vi "NIMS_NS_fir_halfband.vi"(5 "Function name":string, 6 "Line number":i32, 7 "Number of outputs requested":i32, 8 "error in (no error)":errorcluster, 11 "[A]":variant[](array[variant])) -> (0 "error out":errorcluster, 3 "[funct(A)]":variant[](array[variant]))   [LabVIEW 2017]
uses:
  <vilib>/imath/engines/lvmath/Functions/Error Handling/error.ctl
  <instcachedir>/0/NIMS_RunTimeType_From StrictType (excl LVString)_1019F277F0A747EDBCA0F6C52CA54500.lvgen/NIMS_RunTimeType_From StrictType (excl LVString)_1019F277F0A747EDBCA0F6C52CA54500_000.vi
  <instcachedir>/0/NIMS_Get Row Vector_w Error - Matrix_7ECCFA0649AF47C08F6F0C496599EB01.lvgen/NIMS_Get Row Vector_w Error - Matrix_7ECCFA0649AF47C08F6F0C496599EB01_000.vi
  <instcachedir>/0/NIMS_Get Scalar_w Error_1987D997E87247DDAC16EA23A5E9E4FC.lvgen/NIMS_Get Scalar_w Error_1987D997E87247DDAC16EA23A5E9E4FC_003.vi
  <instcachedir>/0/NIMS_Complex To Real_BE01396FDE034E8E94CEBBA1E368668D.lvgen/NIMS_Complex To Real_BE01396FDE034E8E94CEBBA1E368668D_000.vi
  <instcachedir>/0/NIMS_Get Row Vector_w Error - Matrix_7ECCFA0649AF47C08F6F0C496599EB01.lvgen/NIMS_Get Row Vector_w Error - Matrix_7ECCFA0649AF47C08F6F0C496599EB01_001.vi
  <instcachedir>/0/NIMS_RunTimeType_To Numeric_1CBDAFC4EFAD4045A1DE52278D16738D.lvgen/NIMS_RunTimeType_To Numeric_1CBDAFC4EFAD4045A1DE52278D16738D_000.vi
  <instcachedir>/0/NIMS_Get Scalar_w Error_1987D997E87247DDAC16EA23A5E9E4FC.lvgen/NIMS_Get Scalar_w Error_1987D997E87247DDAC16EA23A5E9E4FC_000.vi
  <vilib>/addons/Digital Filter Design/NI_DigFilter_MathScript.lvlib
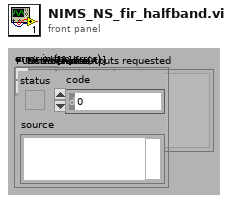
[diagram p1: front panel]
types:
  T1 = typedef "error.ctl" = enum16{"No Error", "Problem", "Input type must not be void", "Incorrect number of parameters", "Function not defined for non-numeric types", "An output variable of the user-defined function is undefined", "Function only defined for character arrays", "Function not defined for boolean, character, or single precision", "Function not defined for complex types", "Not a valid operation", "Inputs must be scalar", "Input matrices are not the same size", "Function only available on RT", "Input matrices must be nonnegative integers of the same type", "Arguments must be non-negative integers less than bitmax", "Number to complement must be less than 2^N", "Bit to get is outside range", "Bit to set is outside range", "Input must be real type ", "At least one parameter must be scalar", "Unable to display plug-in data on RT", "Function not defined for higher dimensional matrices", "Invalid attributes", "Wrong Type of Input Arguments", "Wrong Argument Option", "Invalid file identifier", "Indices must be real positive integers", "The variable is not a matrix data type.", "Number of elements must be the same for indices and values", "You cannot replace elements of a matrix with non-matrix data types.", "Cannot resize a 2D matrix with a linear index", "Unknown variable or symbol", "Indices out of range", "Empty matrix deletion can not be used with two indices", "Number of rows and columns must be the same for indices and values.", "Complex cannot be converted to Boolean", "Char cannot be converted to Boolean", "int64 cannot be converted to Boolean", "uint64 cannot be converted to Boolean", "You cannot convert a Boolean to a character.", "Incompatible input size in 3D surface function", "All rows must have the same number of columns", "Incompatible types", "Invalid matrix dimensions", "Dimension must be 1 or 2", "Base must be an integer between 2 and 36", "Invalid input", "Square matrix required", "Function 'timerstart' must be called before 'timerstop'", "Arguments must be positive real", "Step must not be zero", "Wrong number of input arguments", "Wrong number of output arguments", "Too many index arguments", "Input scalar must be >= 0", "Input scalar must be positive", "Input scalar must not be 0", "Input scalar must be in range [0,1]", "Can't use conditionally defined variable that's undefined", "Input must be a vector", "RT Exec Trace Toolkit not licensed", "Empty vector error", "All elements must be in domain [-1,1]", "All real elements of input vector must be >= 0", "All elements of input vector must be positive", "Values of input vectors are not compatible", "DAQmx not installed", "Input vector must be an increasing vector", "Dereferenced field does not exist within the struct", "A vector or matrix of structures must be indexed before it can be dereferenced", "Lenths of two input vectors are not compatible", "Invalid fieldname", "Empty matrix error", "Cannot use '.' on a type other than Struct", "Unused074", "Data type of the struct's field name is invalid", "Using . to dereference data that is not a struct", "Input struct contains invalid type ", "Size of input matrix is incompatible with input size", "Invalid format specifier", "Could not find field within struct", "Bad permutation array", "Mismatched fieldnames", "ode: User Function could not be opened", "ode: User Function signature does not meet ode requirements", "Unused085", "RunTime: MathScript could not be compiled", "Unknown function", "Only scalars and strings supported", "ode: User Function signature has incorrect number of inputs", "ode:User Function signature has incorrect number of outputs", "Range is too large", "End used without variable", "Function not available (RTE)", "Custom user error", "Arguments must be integers less than bitmax", "Shared library not found", "Header file not found", "Shared library already loaded", "Shared library not loaded", "Shared library function not found", "Shared library string return problem", "Problem calling shared library function", "Problem loading shared library from OS", "Problem parsing shared library header file", "Shared library incompatible types", "Shared library unsupported return type", "Shared library function not exported", "Shared library unsupported input type", "Problem unloading shared library from OS", "Function only available from UI", "Function specified in argument is missing", "An internal error has occurred", "Invalid object", "Invalid property", "Read-only property", "A break command has occurred", "A continue command has occurred", "A return command has occurred", "ode: times parameter invalid", "Function specified in argument has incorrect signature", "Function not found in file", "Reserved keyword cannot be defined as variable", "Reserved keyword cannot be defined as a function or script", "Arguments must be string literals", "Function not supported on this platform", "All columns must have the same number of rows", "Function ignored in RTE warning", "Cannot use : as a parameter that is not a variable", "Output can't be coerced to requested type", "Function not supported on current target", "Variable dependent on an unwired function input", "Unused132", "Unused133", "Unused134", "Unused135", "Unused136", "Unused137", "Unused138", "Unused139", "Global/Persistent must only take constants as arguments.", "Varargin must be last input in the function definition.", "Varargout must be last output in the function definition.", "Invalid output type. Cannot output a cell array of any type other than string.", "Invalid output type. Type is a dynamic struct.", "Invalid output type. Type is a struct that has a field whose type is not known until run-time", "Invalid output type. Type is a struct that has a field which is a plot object.", "MathScript parser DLL missing", "MathScript requires LabVIEW Full", "MathScript license is invalid or missing", "Varargout not supported except in assignments."}
  T2 = typedef "NIMS_CH_character datatype.ctl" = cluster{"Numeric":u8}
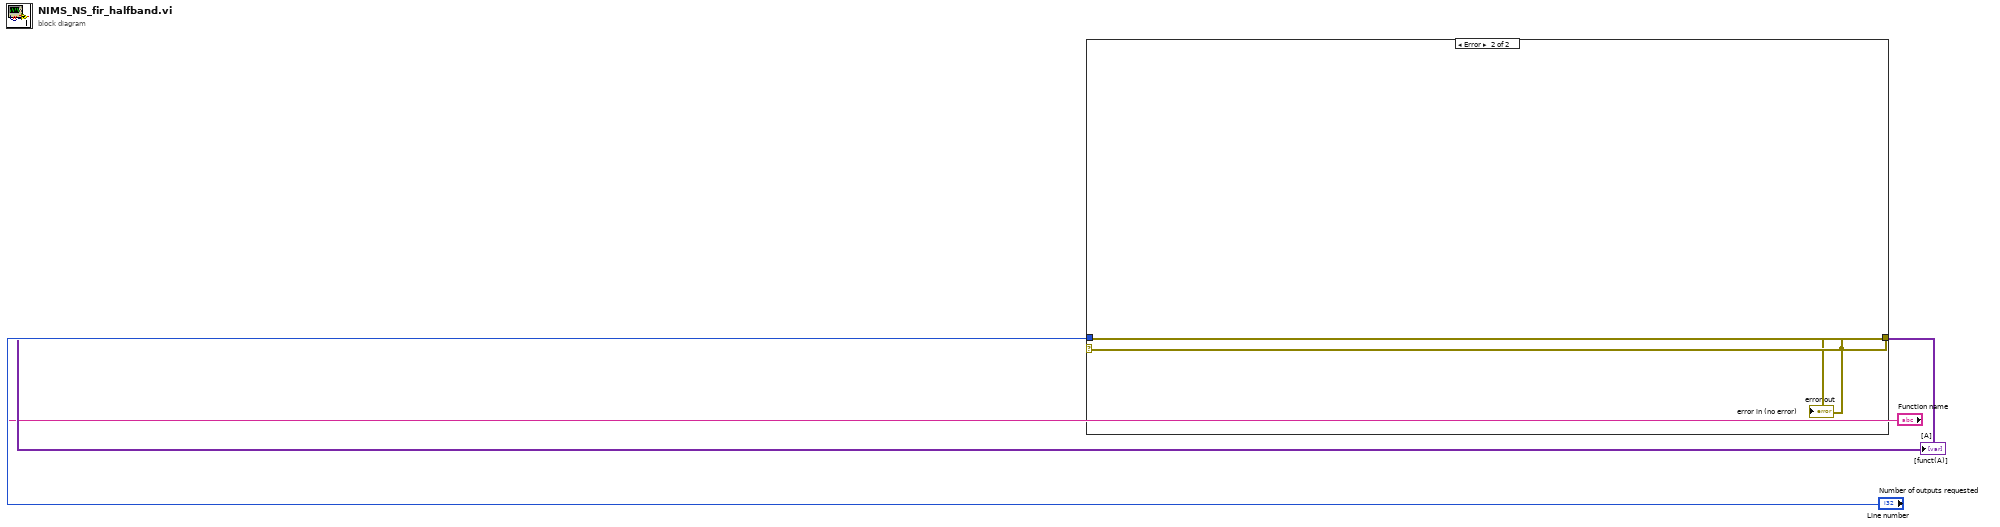
[diagram p0: block diagram]
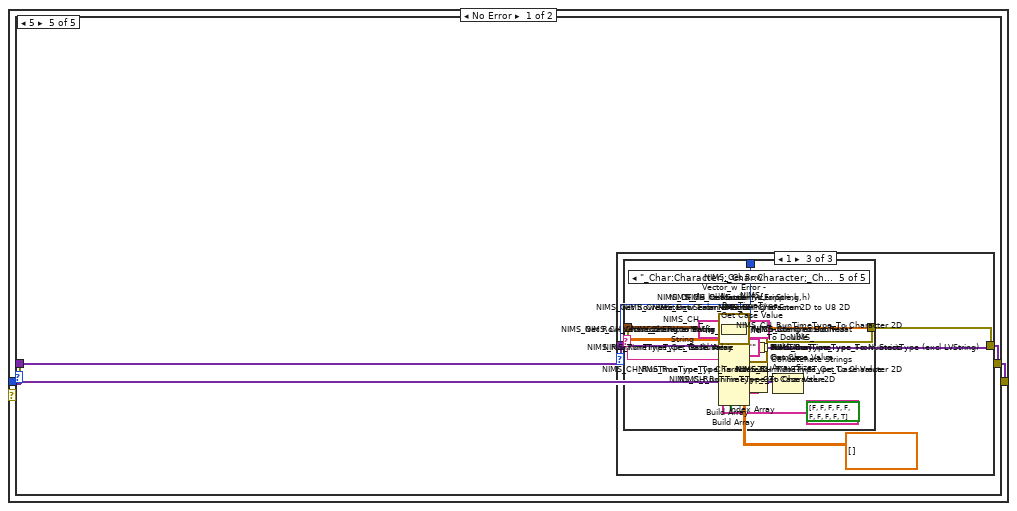
[diagram p2: hidden frame]
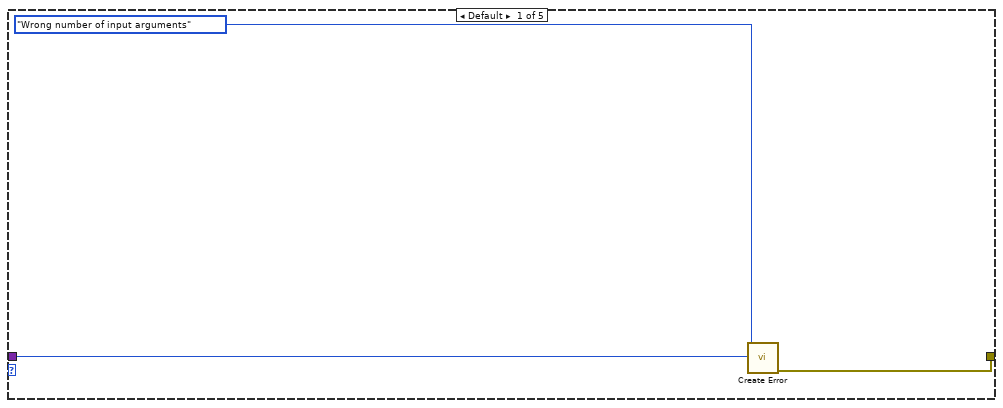
[diagram p3: hidden frame]
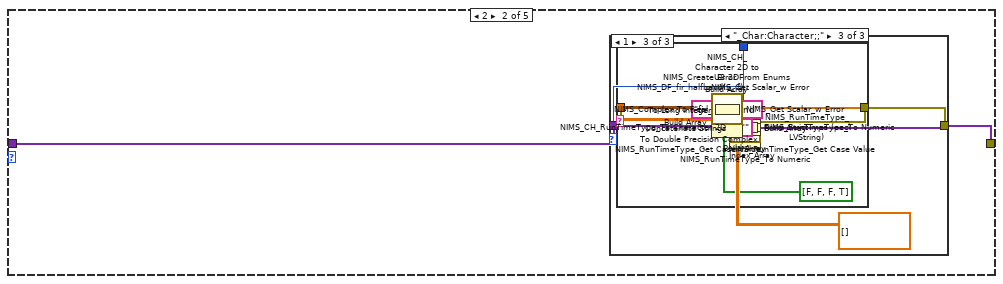
[diagram p4: hidden frame]
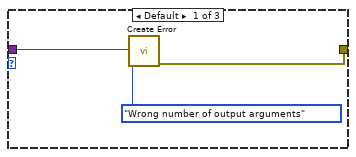
[diagram p5: hidden frame]
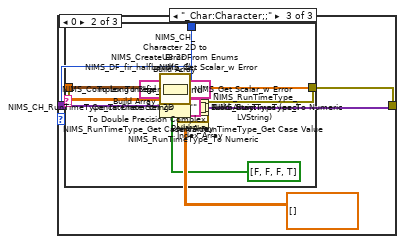
[diagram p6: hidden frame]
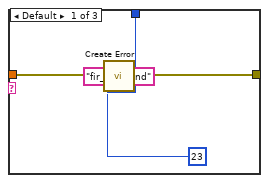
[diagram p7: hidden frame]
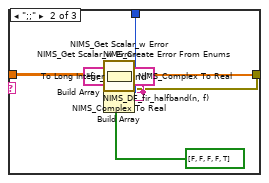
[diagram p8: hidden frame]
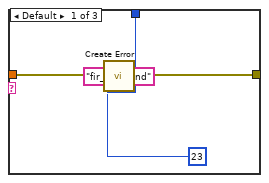
[diagram p9: hidden frame]
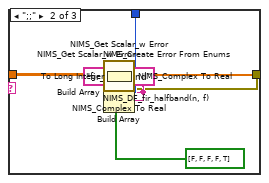
[diagram p10: hidden frame]
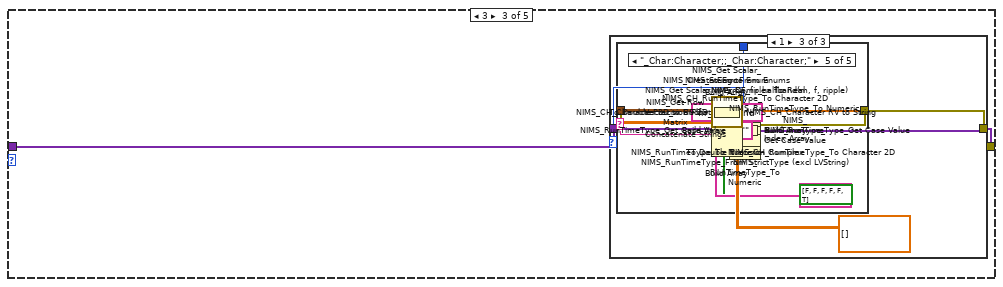
[diagram p11: hidden frame]
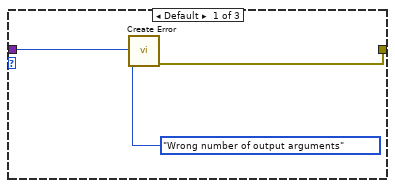
[diagram p12: hidden frame]
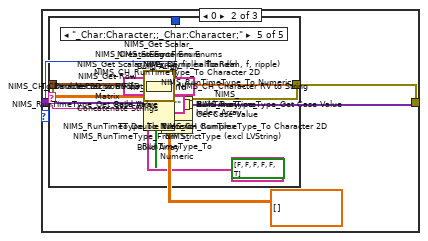
[diagram p13: hidden frame]
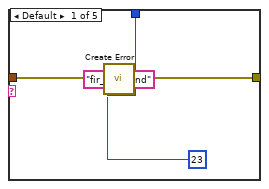
[diagram p14: hidden frame]
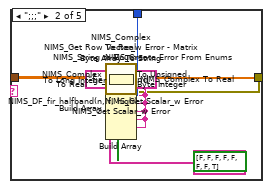
[diagram p15: hidden frame]
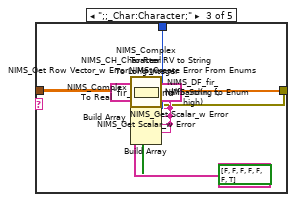
[diagram p16: hidden frame]
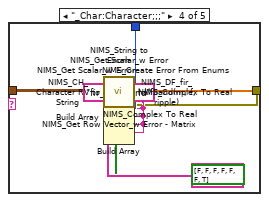
[diagram p17: hidden frame]
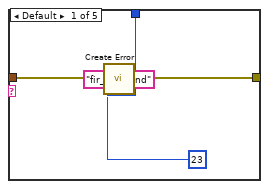
[diagram p18: hidden frame]
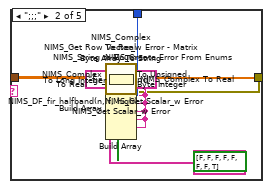
[diagram p19: hidden frame]
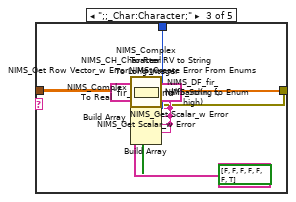
[diagram p20: hidden frame]
diagram:
  n1 = case shown="Error" "error in (no error)" {
    selector: "error in (no error)" -> [_ w1249]
    tunnel: [w15 _] -> w4
    tunnel: [w14 w1249] -> w3
    tunnel: "error in (no error)" -> [w13 _]
    tunnel: "Number of outputs requested" -> [w12 _]
    tunnel: "[A]" -> [w11 _]
    tunnel: "Function name" -> [w10 _]
    tunnel: "Line number" -> [w9 _]
    frame No Error {
      n2 = Array Size(array=w11) -> (size(s)=w8:i32)
      n3 = case shown="5" w8 {
        tunnel: [_ w27 w171 w469 w831] -> w15
        tunnel: w10 -> [w19 w24 w168 w466 w828]
        tunnel: w9 -> [w20 w25 w169 w467 w829]
        tunnel: w13 -> [w17 w23 w167 w465 w827]
        tunnel: [w16 w22 w166 w464 w826] -> w14
        tunnel: w12 -> [_ w21 w165 w463 w825]
        tunnel: w11 -> [_ w26 w170 w468 w830]
        frame Default {
          n4 = call <vilib>:"Create Error.vi"("Function name"=w19, "error in (no error)"=w17, "Error Enum"=error."Wrong number of input arguments", "Line number"=w20) -> ("error out"=w16:errorcluster)  [unwired: 6 in, 1 out]
        }
        frame 2 {
          n5 = case shown="1" w21 {
            tunnel: [_ w33 w99] -> w27
            tunnel: w24 -> [w31 _ _]
            tunnel: w25 -> [w32 w51 w117]
            tunnel: w23 -> [w29 w49 w115]
            tunnel: [w28 w39 w105] -> w22
            tunnel: w26 -> [_ w52 w118]
            frame Default {
              n6 = call <vilib>:"Create Error.vi"("Function name"=w31, "error in (no error)"=w29, "Error Enum"=error."Wrong number of output arguments", "Line number"=w32) -> ("error out"=w28:errorcluster)  [unwired: 6 in, 1 out]
            }
            frame 0 {
              n7 = Index Array(array=w52) -> (element #1=w48:variant, element #2=w43:variant)  [unwired: 2 in]
              n8 = call <vilib>:"NIMS_RunTimeType_Get Case Value.vi"("Data In"=w43) -> ("Case Value"=w40:string)  [unwired: 9 in, 1 out]
              n9 = call-generic <vilib>:"NIMS_RunTimeType_To Numeric.vi"("DataType"=cdb[][] [], "Variant"=w43) -> ("data"=w41:cdb[][])  [unwired: 1 in]
              n10 = call <vilib>:"NIMS_RunTimeType_Get Case Value.vi"("Data In"=w48) -> ("Case Value"=w44:string)  [unwired: 9 in, 1 out]
              n11 = call <vilib>:"NIMS_CH_RunTimeType_To Character 2D.vi"("Variant"=w48) -> ("data"=w45:T2[][])  [unwired: 1 in]
              n12 = call-generic <vilib>:"NIMS_RunTimeType_To Numeric.vi"("DataType"=cdb[][] [], "Variant"=w48) -> ("data"=w46:cdb[][])  [unwired: 1 in]
              n13 = Concatenate Strings(w44, w40) -> (w50:string)
              n14 = case shown="\"_Char:Character;;\"" w50 {
                tunnel: w49 -> [w54 w63 w84]
                tunnel: [_ w58 w79] -> w38
                tunnel: [w53 w59 w80] -> w39
                tunnel: w46 -> [_ w77 _]
                tunnel: w45 -> [_ _ w97]
                tunnel: w41 -> [_ w73 w93]
                tunnel: w51 -> [w57 w66 w87]
                frame Default {
                  n15 = call <vilib>:"Create Error.vi"("Function name"="fir_halfband", "error in (no error)"=w54, "Error Enum"=23, "Line number"=w57) -> ("error out"=w53:errorcluster)  [unwired: 6 in, 1 out]
                }
                frame ";;" {
                  w61 = "fir_halfband"
                  n16 = call-generic <vilib>:"NIMS_Complex To Real.vi"("A"=w73) -> ("Error Enum"=w69:T1, "Real(A)"=w72:dbl[][])  [unwired: 8 in, 1 out]
                  n17 = call-generic <vilib>:"NIMS_Get Scalar_w Error.vi"("A"=w72) -> ("Error Enum"=w68:T1, "Scalar"=w74:dbl)  [unwired: 8 in, 1 out]
                  n18 = call-generic <vilib>:"NIMS_Complex To Real.vi"("A"=w77) -> ("Error Enum"=w71:T1, "Real(A)"=w76:dbl[][])  [unwired: 8 in, 1 out]
                  n19 = To Long Integer(number=w76) -> (32bit integer=w75:i32[][])
                  n20 = call-generic <vilib>:"NIMS_Get Scalar_w Error.vi"("A"=w75) -> ("Error Enum"=w70:T1, "Scalar"=w78:i32)  [unwired: 8 in, 1 out]
                  n21 = call <vilib>:"NIMS_DF_fir_halfband(n, f).vi"("f"=w74, "n"=w78) -> ("error"=w67:i32, "b"=w58:dbl[])  [unwired: 8 in]
                  n22 = Build Array(w61, w61, w61, w61, "fir_halfband") -> (w64:string[])
                  n23 = Build Array(w71, w70, w69, w68, w67) -> (w65:i32[])
                  n24 = call <vilib>:"NIMS_Create Error From Enums.vi"("Error Code"=bool[] [FALSE, FALSE, FALSE, FALSE, TRUE], "error in (no error)"=w63, "Line no"=w66, "Error Enums"=w65, "Function names"=w64) -> ("error out"=w59:errorcluster)  [unwired: 6 in]
                }
                frame "_Char:Character;;" {
                  w82 = "fir_halfband"
                  n25 = call-generic <vilib>:"NIMS_Complex To Real.vi"("A"=w93) -> ("Error Enum"=w90:T1, "Real(A)"=w92:dbl[][])  [unwired: 8 in, 1 out]
                  n26 = call-generic <vilib>:"NIMS_Get Scalar_w Error.vi"("A"=w92) -> ("Error Enum"=w89:T1, "Scalar"=w94:dbl)  [unwired: 8 in, 1 out]
                  n27 = call <vilib>:"NIMS_CH_Character 2D to U8 2D.vi"("Character 2D array"=w97) -> ("U8 2D array"=w96:u8[][])  [unwired: 10 in]
                  n28 = To Long Integer(number=w96) -> (32bit integer=w95:i32[][])
                  n29 = call-generic <vilib>:"NIMS_Get Scalar_w Error.vi"("A"=w95) -> ("Error Enum"=w91:T1, "Scalar"=w98:i32)  [unwired: 8 in, 1 out]
                  n30 = call <vilib>:"NIMS_DF_fir_halfband(n, f).vi"("f"=w94, "n"=w98) -> ("error"=w88:i32, "b"=w79:dbl[])  [unwired: 8 in]
                  n31 = Build Array(w82, w82, w82, "fir_halfband") -> (w85:string[])
                  n32 = Build Array(w91, w90, w89, w88) -> (w86:i32[])
                  n33 = call <vilib>:"NIMS_Create Error From Enums.vi"("Error Code"=bool[] [FALSE, FALSE, FALSE, TRUE], "error in (no error)"=w84, "Line no"=w87, "Error Enums"=w86, "Function names"=w85) -> ("error out"=w80:errorcluster)  [unwired: 6 in]
                }
              }
              n34 = Build Array(w38) -> (w37:dbl[][])
              n35 = To Double Precision Complex(1:w37) -> (0:w36:cdb[][])
              n36 = call-generic <vilib>:"NIMS_RunTimeType_From StrictType (excl LVString).vi"("Plug-In Name"="", "Data In"=w36) -> ("Data Out"=w34:variant)  [unwired: 2 in]
              n37 = Build Array(w34) -> (w33:variant[])
            }
            frame 1 {
              n38 = Index Array(array=w118) -> (element #1=w114:variant, element #2=w109:variant)  [unwired: 2 in]
              n39 = call <vilib>:"NIMS_RunTimeType_Get Case Value.vi"("Data In"=w109) -> ("Case Value"=w106:string)  [unwired: 9 in, 1 out]
              n40 = call-generic <vilib>:"NIMS_RunTimeType_To Numeric.vi"("DataType"=cdb[][] [], "Variant"=w109) -> ("data"=w107:cdb[][])  [unwired: 1 in]
              n41 = call <vilib>:"NIMS_RunTimeType_Get Case Value.vi"("Data In"=w114) -> ("Case Value"=w110:string)  [unwired: 9 in, 1 out]
              n42 = call <vilib>:"NIMS_CH_RunTimeType_To Character 2D.vi"("Variant"=w114) -> ("data"=w111:T2[][])  [unwired: 1 in]
              n43 = call-generic <vilib>:"NIMS_RunTimeType_To Numeric.vi"("DataType"=cdb[][] [], "Variant"=w114) -> ("data"=w112:cdb[][])  [unwired: 1 in]
              n44 = Concatenate Strings(w110, w106) -> (w116:string)
              n45 = case shown="\"_Char:Character;;\"" w116 {
                tunnel: w115 -> [w120 w129 w150]
                tunnel: [_ w124 w145] -> w104
                tunnel: [w119 w125 w146] -> w105
                tunnel: w112 -> [_ w143 _]
                tunnel: w111 -> [_ _ w163]
                tunnel: w107 -> [_ w139 w159]
                tunnel: w117 -> [w123 w132 w153]
                frame Default {
                  n46 = call <vilib>:"Create Error.vi"("Function name"="fir_halfband", "error in (no error)"=w120, "Error Enum"=23, "Line number"=w123) -> ("error out"=w119:errorcluster)  [unwired: 6 in, 1 out]
                }
                frame ";;" {
                  w127 = "fir_halfband"
                  n47 = call-generic <vilib>:"NIMS_Complex To Real.vi"("A"=w139) -> ("Error Enum"=w135:T1, "Real(A)"=w138:dbl[][])  [unwired: 8 in, 1 out]
                  n48 = call-generic <vilib>:"NIMS_Get Scalar_w Error.vi"("A"=w138) -> ("Error Enum"=w134:T1, "Scalar"=w140:dbl)  [unwired: 8 in, 1 out]
                  n49 = call-generic <vilib>:"NIMS_Complex To Real.vi"("A"=w143) -> ("Error Enum"=w137:T1, "Real(A)"=w142:dbl[][])  [unwired: 8 in, 1 out]
                  n50 = To Long Integer(number=w142) -> (32bit integer=w141:i32[][])
                  n51 = call-generic <vilib>:"NIMS_Get Scalar_w Error.vi"("A"=w141) -> ("Error Enum"=w136:T1, "Scalar"=w144:i32)  [unwired: 8 in, 1 out]
                  n52 = call <vilib>:"NIMS_DF_fir_halfband(n, f).vi"("f"=w140, "n"=w144) -> ("error"=w133:i32, "b"=w124:dbl[])  [unwired: 8 in]
                  n53 = Build Array(w127, w127, w127, w127, "fir_halfband") -> (w130:string[])
                  n54 = Build Array(w137, w136, w135, w134, w133) -> (w131:i32[])
                  n55 = call <vilib>:"NIMS_Create Error From Enums.vi"("Error Code"=bool[] [FALSE, FALSE, FALSE, FALSE, TRUE], "error in (no error)"=w129, "Line no"=w132, "Error Enums"=w131, "Function names"=w130) -> ("error out"=w125:errorcluster)  [unwired: 6 in]
                }
                frame "_Char:Character;;" {
                  w148 = "fir_halfband"
                  n56 = call-generic <vilib>:"NIMS_Complex To Real.vi"("A"=w159) -> ("Error Enum"=w156:T1, "Real(A)"=w158:dbl[][])  [unwired: 8 in, 1 out]
                  n57 = call-generic <vilib>:"NIMS_Get Scalar_w Error.vi"("A"=w158) -> ("Error Enum"=w155:T1, "Scalar"=w160:dbl)  [unwired: 8 in, 1 out]
                  n58 = call <vilib>:"NIMS_CH_Character 2D to U8 2D.vi"("Character 2D array"=w163) -> ("U8 2D array"=w162:u8[][])  [unwired: 10 in]
                  n59 = To Long Integer(number=w162) -> (32bit integer=w161:i32[][])
                  n60 = call-generic <vilib>:"NIMS_Get Scalar_w Error.vi"("A"=w161) -> ("Error Enum"=w157:T1, "Scalar"=w164:i32)  [unwired: 8 in, 1 out]
                  n61 = call <vilib>:"NIMS_DF_fir_halfband(n, f).vi"("f"=w160, "n"=w164) -> ("error"=w154:i32, "b"=w145:dbl[])  [unwired: 8 in]
                  n62 = Build Array(w148, w148, w148, "fir_halfband") -> (w151:string[])
                  n63 = Build Array(w157, w156, w155, w154) -> (w152:i32[])
                  n64 = call <vilib>:"NIMS_Create Error From Enums.vi"("Error Code"=bool[] [FALSE, FALSE, FALSE, TRUE], "error in (no error)"=w150, "Line no"=w153, "Error Enums"=w152, "Function names"=w151) -> ("error out"=w146:errorcluster)  [unwired: 6 in]
                }
              }
              n65 = Build Array(w104) -> (w103:dbl[][])
              n66 = To Double Precision Complex(1:w103) -> (0:w102:cdb[][])
              n67 = call-generic <vilib>:"NIMS_RunTimeType_From StrictType (excl LVString).vi"("Plug-In Name"="", "Data In"=w102) -> ("Data Out"=w100:variant)  [unwired: 2 in]
              n68 = Build Array(w100) -> (w99:variant[])
            }
          }
        }
        frame 3 {
          n69 = case shown="1" w165 {
            tunnel: [_ w177 w320] -> w171
            tunnel: w168 -> [w175 _ _]
            tunnel: w169 -> [w176 w200 w343]
            tunnel: w167 -> [w173 w198 w341]
            tunnel: [w172 w183 w326] -> w166
            tunnel: w170 -> [_ w201 w344]
            frame Default {
              n70 = call <vilib>:"Create Error.vi"("Function name"=w175, "error in (no error)"=w173, "Error Enum"=error."Wrong number of output arguments", "Line number"=w176) -> ("error out"=w172:errorcluster)  [unwired: 6 in, 1 out]
            }
            frame 0 {
              n71 = Index Array(array=w201) -> (element #1=w197:variant, element #2=w192:variant, element #3=w188:variant)  [unwired: 3 in]
              n72 = call <vilib>:"NIMS_RunTimeType_Get Case Value.vi"("Data In"=w188) -> ("Case Value"=w184:string)  [unwired: 9 in, 1 out]
              n73 = call <vilib>:"NIMS_CH_RunTimeType_To Character 2D.vi"("Variant"=w188) -> ("data"=w185:T2[][])  [unwired: 1 in]
              n74 = call-generic <vilib>:"NIMS_RunTimeType_To Numeric.vi"("DataType"=cdb[][] [], "Variant"=w188) -> ("data"=w186:cdb[][])  [unwired: 1 in]
              n75 = call <vilib>:"NIMS_RunTimeType_Get Case Value.vi"("Data In"=w192) -> ("Case Value"=w189:string)  [unwired: 9 in, 1 out]
              n76 = call-generic <vilib>:"NIMS_RunTimeType_To Numeric.vi"("DataType"=cdb[][] [], "Variant"=w192) -> ("data"=w190:cdb[][])  [unwired: 1 in]
              n77 = call <vilib>:"NIMS_RunTimeType_Get Case Value.vi"("Data In"=w197) -> ("Case Value"=w193:string)  [unwired: 9 in, 1 out]
              n78 = call <vilib>:"NIMS_CH_RunTimeType_To Character 2D.vi"("Variant"=w197) -> ("data"=w194:T2[][])  [unwired: 1 in]
              n79 = call-generic <vilib>:"NIMS_RunTimeType_To Numeric.vi"("DataType"=cdb[][] [], "Variant"=w197) -> ("data"=w195:cdb[][])  [unwired: 1 in]
              n80 = Concatenate Strings(w193, w189, w184) -> (w199:string)
              n81 = case shown="\"_Char:Character;;_Char:Character;\"" w199 {
                tunnel: w198 -> [w203 w212 w243 w271 w298]
                tunnel: [_ w207 w238 w266 w293] -> w182
                tunnel: [w202 w208 w239 w267 w294] -> w183
                tunnel: w195 -> [_ w236 w264 _ _]
                tunnel: w194 -> [_ _ _ w290 w317]
                tunnel: w190 -> [_ w232 w260 w286 w313]
                tunnel: w186 -> [_ w228 _ w283 _]
                tunnel: w185 -> [_ _ w256 _ w310]
                tunnel: w200 -> [w206 w215 w246 w274 w301]
                frame Default {
                  n82 = call <vilib>:"Create Error.vi"("Function name"="fir_halfband", "error in (no error)"=w203, "Error Enum"=23, "Line number"=w206) -> ("error out"=w202:errorcluster)  [unwired: 6 in, 1 out]
                }
                frame ";;;" {
                  w210 = "fir_halfband"
                  n83 = call-generic <vilib>:"NIMS_Complex To Real.vi"("A"=w228) -> ("Error Enum"=w219:T1, "Real(A)"=w227:dbl[][])  [unwired: 8 in, 1 out]
                  n84 = To Unsigned Byte Integer(number=w227) -> (unsigned 8bit integer=w226:u8[][])
                  n85 = call-generic <vilib>:"NIMS_Get Row Vector_w Error - Matrix.vi"("A"=w226) -> ("Error Enum"=w218:T1, "Row Vector"=w225:u8[])  [unwired: 8 in, 1 out]
                  n86 = Byte Array To String(unsigned byte array=w225) -> (string=w229:string)
                  n87 = call <vilib>:"NIMS_String to Enum.vi"("Input String"=w229, "Enum choices"=string[] ["high"] ("Enum Options")) -> ("Error Enum"=w217:T1, "Enum Index"=w230:i32)  [unwired: 8 in]
                  n88 = call-generic <vilib>:"NIMS_Complex To Real.vi"("A"=w232) -> ("Error Enum"=w221:T1, "Real(A)"=w231:dbl[][])  [unwired: 8 in, 1 out]
                  n89 = call-generic <vilib>:"NIMS_Get Scalar_w Error.vi"("A"=w231) -> ("Error Enum"=w220:T1, "Scalar"=w233:dbl)  [unwired: 8 in, 1 out]
                  n90 = call-generic <vilib>:"NIMS_Complex To Real.vi"("A"=w236) -> ("Error Enum"=w223:T1, "Real(A)"=w235:dbl[][])  [unwired: 8 in, 1 out]
                  n91 = To Long Integer(number=w235) -> (32bit integer=w234:i32[][])
                  n92 = call-generic <vilib>:"NIMS_Get Scalar_w Error.vi"("A"=w234) -> ("Error Enum"=w222:T1, "Scalar"=w237:i32)  [unwired: 8 in, 1 out]
                  n93 = call <vilib>:"NIMS_DF_fir_halfband(n, f, high).vi"("type"=w230, "f"=w233, "n"=w237) -> ("error"=w216:i32, "b"=w207:dbl[])  [unwired: 7 in]
                  n94 = Build Array(w210, w210, w210, w210, w210, w210, w210, "fir_halfband") -> (w213:string[])
                  n95 = Build Array(w223, w222, w221, w220, w219, w218, w217, w216) -> (w214:i32[])
                  n96 = call <vilib>:"NIMS_Create Error From Enums.vi"("Error Code"=bool[] [FALSE, FALSE, FALSE, FALSE, FALSE, FALSE, FALSE, TRUE], "error in (no error)"=w212, "Line no"=w215, "Error Enums"=w214, "Function names"=w213) -> ("error out"=w208:errorcluster)  [unwired: 6 in]
                }
                frame ";;_Char:Character;" {
                  w241 = "fir_halfband"
                  n97 = call-generic <vilib>:"NIMS_Get Row Vector_w Error - Matrix.vi"("A"=w256) -> ("Error Enum"=w249:T1, "Row Vector"=w255:T2[])  [unwired: 8 in, 1 out]
                  n98 = call <vilib>:"NIMS_CH_Character RV to String.vi"("Character array"=w255) -> ("String"=w257:string)  [unwired: 10 in]
                  n99 = call <vilib>:"NIMS_String to Enum.vi"("Input String"=w257, "Enum choices"=string[] ["high"] ("Enum Options")) -> ("Error Enum"=w248:T1, "Enum Index"=w258:i32)  [unwired: 8 in]
                  n100 = call-generic <vilib>:"NIMS_Complex To Real.vi"("A"=w260) -> ("Error Enum"=w251:T1, "Real(A)"=w259:dbl[][])  [unwired: 8 in, 1 out]
                  n101 = call-generic <vilib>:"NIMS_Get Scalar_w Error.vi"("A"=w259) -> ("Error Enum"=w250:T1, "Scalar"=w261:dbl)  [unwired: 8 in, 1 out]
                  n102 = call-generic <vilib>:"NIMS_Complex To Real.vi"("A"=w264) -> ("Error Enum"=w253:T1, "Real(A)"=w263:dbl[][])  [unwired: 8 in, 1 out]
                  n103 = To Long Integer(number=w263) -> (32bit integer=w262:i32[][])
                  n104 = call-generic <vilib>:"NIMS_Get Scalar_w Error.vi"("A"=w262) -> ("Error Enum"=w252:T1, "Scalar"=w265:i32)  [unwired: 8 in, 1 out]
                  n105 = call <vilib>:"NIMS_DF_fir_halfband(n, f, high).vi"("type"=w258, "f"=w261, "n"=w265) -> ("error"=w247:i32, "b"=w238:dbl[])  [unwired: 7 in]
                  n106 = Build Array(w241, w241, w241, w241, w241, w241, "fir_halfband") -> (w244:string[])
                  n107 = Build Array(w253, w252, w251, w250, w249, w248, w247) -> (w245:i32[])
                  n108 = call <vilib>:"NIMS_Create Error From Enums.vi"("Error Code"=bool[] [FALSE, FALSE, FALSE, FALSE, FALSE, FALSE, TRUE], "error in (no error)"=w243, "Line no"=w246, "Error Enums"=w245, "Function names"=w244) -> ("error out"=w239:errorcluster)  [unwired: 6 in]
                }
                frame "_Char:Character;;;" {
                  w269 = "fir_halfband"
                  n109 = call-generic <vilib>:"NIMS_Complex To Real.vi"("A"=w283) -> ("Error Enum"=w277:T1, "Real(A)"=w282:dbl[][])  [unwired: 8 in, 1 out]
                  n110 = call-generic <vilib>:"NIMS_Get Scalar_w Error.vi"("A"=w282) -> ("Error Enum"=w276:T1, "Scalar"=w284:dbl)  [unwired: 8 in, 1 out]
                  n111 = call-generic <vilib>:"NIMS_Complex To Real.vi"("A"=w286) -> ("Error Enum"=w279:T1, "Real(A)"=w285:dbl[][])  [unwired: 8 in, 1 out]
                  n112 = call-generic <vilib>:"NIMS_Get Scalar_w Error.vi"("A"=w285) -> ("Error Enum"=w278:T1, "Scalar"=w287:dbl)  [unwired: 8 in, 1 out]
                  n113 = call-generic <vilib>:"NIMS_Get Row Vector_w Error - Matrix.vi"("A"=w290) -> ("Error Enum"=w281:T1, "Row Vector"=w289:T2[])  [unwired: 8 in, 1 out]
                  n114 = call <vilib>:"NIMS_CH_Character RV to String.vi"("Character array"=w289) -> ("String"=w291:string)  [unwired: 10 in]
                  n115 = call <vilib>:"NIMS_String to Enum.vi"("Input String"=w291, "Enum choices"=string[] ["minorder"] ("Enum Options")) -> ("Error Enum"=w280:T1, "Enum Index"=w292:i32)  [unwired: 8 in]
                  n116 = call <vilib>:"NIMS_DF_fir_halfband(m, f, ripple).vi"("ripple"=w284, "f"=w287, "flag"=w292) -> ("error"=w275:i32, "b"=w266:dbl[])  [unwired: 7 in]
                  n117 = Build Array(w269, w269, w269, w269, w269, w269, "fir_halfband") -> (w272:string[])
                  n118 = Build Array(w281, w280, w279, w278, w277, w276, w275) -> (w273:i32[])
                  n119 = call <vilib>:"NIMS_Create Error From Enums.vi"("Error Code"=bool[] [FALSE, FALSE, FALSE, FALSE, FALSE, FALSE, TRUE], "error in (no error)"=w271, "Line no"=w274, "Error Enums"=w273, "Function names"=w272) -> ("error out"=w267:errorcluster)  [unwired: 6 in]
                }
                frame "_Char:Character;;_Char:Character;" {
                  w296 = "fir_halfband"
                  n120 = call <vilib>:"NIMS_CH_Character 2D to U8 2D.vi"("Character 2D array"=w310) -> ("U8 2D array"=w309:u8[][])  [unwired: 10 in]
                  n121 = To Double Precision Float(number=w309) -> (double precision float=w308:dbl[][])
                  n122 = call-generic <vilib>:"NIMS_Get Scalar_w Error.vi"("A"=w308) -> ("Error Enum"=w303:T1, "Scalar"=w311:dbl)  [unwired: 8 in, 1 out]
                  n123 = call-generic <vilib>:"NIMS_Complex To Real.vi"("A"=w313) -> ("Error Enum"=w305:T1, "Real(A)"=w312:dbl[][])  [unwired: 8 in, 1 out]
                  n124 = call-generic <vilib>:"NIMS_Get Scalar_w Error.vi"("A"=w312) -> ("Error Enum"=w304:T1, "Scalar"=w314:dbl)  [unwired: 8 in, 1 out]
                  n125 = call-generic <vilib>:"NIMS_Get Row Vector_w Error - Matrix.vi"("A"=w317) -> ("Error Enum"=w307:T1, "Row Vector"=w316:T2[])  [unwired: 8 in, 1 out]
                  n126 = call <vilib>:"NIMS_CH_Character RV to String.vi"("Character array"=w316) -> ("String"=w318:string)  [unwired: 10 in]
                  n127 = call <vilib>:"NIMS_String to Enum.vi"("Input String"=w318, "Enum choices"=string[] ["minorder"] ("Enum Options")) -> ("Error Enum"=w306:T1, "Enum Index"=w319:i32)  [unwired: 8 in]
                  n128 = call <vilib>:"NIMS_DF_fir_halfband(m, f, ripple).vi"("ripple"=w311, "f"=w314, "flag"=w319) -> ("error"=w302:i32, "b"=w293:dbl[])  [unwired: 7 in]
                  n129 = Build Array(w296, w296, w296, w296, w296, "fir_halfband") -> (w299:string[])
                  n130 = Build Array(w307, w306, w305, w304, w303, w302) -> (w300:i32[])
                  n131 = call <vilib>:"NIMS_Create Error From Enums.vi"("Error Code"=bool[] [FALSE, FALSE, FALSE, FALSE, FALSE, TRUE], "error in (no error)"=w298, "Line no"=w301, "Error Enums"=w300, "Function names"=w299) -> ("error out"=w294:errorcluster)  [unwired: 6 in]
                }
              }
              n132 = Build Array(w182) -> (w181:dbl[][])
              n133 = To Double Precision Complex(1:w181) -> (0:w180:cdb[][])
              n134 = call-generic <vilib>:"NIMS_RunTimeType_From StrictType (excl LVString).vi"("Plug-In Name"="", "Data In"=w180) -> ("Data Out"=w178:variant)  [unwired: 2 in]
              n135 = Build Array(w178) -> (w177:variant[])
            }
            frame 1 {
              n136 = Index Array(array=w344) -> (element #1=w340:variant, element #2=w335:variant, element #3=w331:variant)  [unwired: 3 in]
              n137 = call <vilib>:"NIMS_RunTimeType_Get Case Value.vi"("Data In"=w331) -> ("Case Value"=w327:string)  [unwired: 9 in, 1 out]
              n138 = call <vilib>:"NIMS_CH_RunTimeType_To Character 2D.vi"("Variant"=w331) -> ("data"=w328:T2[][])  [unwired: 1 in]
              n139 = call-generic <vilib>:"NIMS_RunTimeType_To Numeric.vi"("DataType"=cdb[][] [], "Variant"=w331) -> ("data"=w329:cdb[][])  [unwired: 1 in]
              n140 = call <vilib>:"NIMS_RunTimeType_Get Case Value.vi"("Data In"=w335) -> ("Case Value"=w332:string)  [unwired: 9 in, 1 out]
              n141 = call-generic <vilib>:"NIMS_RunTimeType_To Numeric.vi"("DataType"=cdb[][] [], "Variant"=w335) -> ("data"=w333:cdb[][])  [unwired: 1 in]
              n142 = call <vilib>:"NIMS_RunTimeType_Get Case Value.vi"("Data In"=w340) -> ("Case Value"=w336:string)  [unwired: 9 in, 1 out]
              n143 = call <vilib>:"NIMS_CH_RunTimeType_To Character 2D.vi"("Variant"=w340) -> ("data"=w337:T2[][])  [unwired: 1 in]
              n144 = call-generic <vilib>:"NIMS_RunTimeType_To Numeric.vi"("DataType"=cdb[][] [], "Variant"=w340) -> ("data"=w338:cdb[][])  [unwired: 1 in]
              n145 = Concatenate Strings(w336, w332, w327) -> (w342:string)
              n146 = case shown="\"_Char:Character;;_Char:Character;\"" w342 {
                tunnel: w341 -> [w346 w355 w386 w414 w441]
                tunnel: [_ w350 w381 w409 w436] -> w325
                tunnel: [w345 w351 w382 w410 w437] -> w326
                tunnel: w338 -> [_ w379 w407 _ _]
                tunnel: w337 -> [_ _ _ w433 w460]
                tunnel: w333 -> [_ w375 w403 w429 w456]
                tunnel: w329 -> [_ w371 _ w426 _]
                tunnel: w328 -> [_ _ w399 _ w453]
                tunnel: w343 -> [w349 w358 w389 w417 w444]
                frame Default {
                  n147 = call <vilib>:"Create Error.vi"("Function name"="fir_halfband", "error in (no error)"=w346, "Error Enum"=23, "Line number"=w349) -> ("error out"=w345:errorcluster)  [unwired: 6 in, 1 out]
                }
                frame ";;;" {
                  w353 = "fir_halfband"
                  n148 = call-generic <vilib>:"NIMS_Complex To Real.vi"("A"=w371) -> ("Error Enum"=w362:T1, "Real(A)"=w370:dbl[][])  [unwired: 8 in, 1 out]
                  n149 = To Unsigned Byte Integer(number=w370) -> (unsigned 8bit integer=w369:u8[][])
                  n150 = call-generic <vilib>:"NIMS_Get Row Vector_w Error - Matrix.vi"("A"=w369) -> ("Error Enum"=w361:T1, "Row Vector"=w368:u8[])  [unwired: 8 in, 1 out]
                  n151 = Byte Array To String(unsigned byte array=w368) -> (string=w372:string)
                  n152 = call <vilib>:"NIMS_String to Enum.vi"("Input String"=w372, "Enum choices"=string[] ["high"] ("Enum Options")) -> ("Error Enum"=w360:T1, "Enum Index"=w373:i32)  [unwired: 8 in]
                  n153 = call-generic <vilib>:"NIMS_Complex To Real.vi"("A"=w375) -> ("Error Enum"=w364:T1, "Real(A)"=w374:dbl[][])  [unwired: 8 in, 1 out]
                  n154 = call-generic <vilib>:"NIMS_Get Scalar_w Error.vi"("A"=w374) -> ("Error Enum"=w363:T1, "Scalar"=w376:dbl)  [unwired: 8 in, 1 out]
                  n155 = call-generic <vilib>:"NIMS_Complex To Real.vi"("A"=w379) -> ("Error Enum"=w366:T1, "Real(A)"=w378:dbl[][])  [unwired: 8 in, 1 out]
                  n156 = To Long Integer(number=w378) -> (32bit integer=w377:i32[][])
                  n157 = call-generic <vilib>:"NIMS_Get Scalar_w Error.vi"("A"=w377) -> ("Error Enum"=w365:T1, "Scalar"=w380:i32)  [unwired: 8 in, 1 out]
                  n158 = call <vilib>:"NIMS_DF_fir_halfband(n, f, high).vi"("type"=w373, "f"=w376, "n"=w380) -> ("error"=w359:i32, "b"=w350:dbl[])  [unwired: 7 in]
                  n159 = Build Array(w353, w353, w353, w353, w353, w353, w353, "fir_halfband") -> (w356:string[])
                  n160 = Build Array(w366, w365, w364, w363, w362, w361, w360, w359) -> (w357:i32[])
                  n161 = call <vilib>:"NIMS_Create Error From Enums.vi"("Error Code"=bool[] [FALSE, FALSE, FALSE, FALSE, FALSE, FALSE, FALSE, TRUE], "error in (no error)"=w355, "Line no"=w358, "Error Enums"=w357, "Function names"=w356) -> ("error out"=w351:errorcluster)  [unwired: 6 in]
                }
                frame ";;_Char:Character;" {
                  w384 = "fir_halfband"
                  n162 = call-generic <vilib>:"NIMS_Get Row Vector_w Error - Matrix.vi"("A"=w399) -> ("Error Enum"=w392:T1, "Row Vector"=w398:T2[])  [unwired: 8 in, 1 out]
                  n163 = call <vilib>:"NIMS_CH_Character RV to String.vi"("Character array"=w398) -> ("String"=w400:string)  [unwired: 10 in]
                  n164 = call <vilib>:"NIMS_String to Enum.vi"("Input String"=w400, "Enum choices"=string[] ["high"] ("Enum Options")) -> ("Error Enum"=w391:T1, "Enum Index"=w401:i32)  [unwired: 8 in]
                  n165 = call-generic <vilib>:"NIMS_Complex To Real.vi"("A"=w403) -> ("Error Enum"=w394:T1, "Real(A)"=w402:dbl[][])  [unwired: 8 in, 1 out]
                  n166 = call-generic <vilib>:"NIMS_Get Scalar_w Error.vi"("A"=w402) -> ("Error Enum"=w393:T1, "Scalar"=w404:dbl)  [unwired: 8 in, 1 out]
                  n167 = call-generic <vilib>:"NIMS_Complex To Real.vi"("A"=w407) -> ("Error Enum"=w396:T1, "Real(A)"=w406:dbl[][])  [unwired: 8 in, 1 out]
                  n168 = To Long Integer(number=w406) -> (32bit integer=w405:i32[][])
                  n169 = call-generic <vilib>:"NIMS_Get Scalar_w Error.vi"("A"=w405) -> ("Error Enum"=w395:T1, "Scalar"=w408:i32)  [unwired: 8 in, 1 out]
                  n170 = call <vilib>:"NIMS_DF_fir_halfband(n, f, high).vi"("type"=w401, "f"=w404, "n"=w408) -> ("error"=w390:i32, "b"=w381:dbl[])  [unwired: 7 in]
                  n171 = Build Array(w384, w384, w384, w384, w384, w384, "fir_halfband") -> (w387:string[])
                  n172 = Build Array(w396, w395, w394, w393, w392, w391, w390) -> (w388:i32[])
                  n173 = call <vilib>:"NIMS_Create Error From Enums.vi"("Error Code"=bool[] [FALSE, FALSE, FALSE, FALSE, FALSE, FALSE, TRUE], "error in (no error)"=w386, "Line no"=w389, "Error Enums"=w388, "Function names"=w387) -> ("error out"=w382:errorcluster)  [unwired: 6 in]
                }
                frame "_Char:Character;;;" {
                  w412 = "fir_halfband"
                  n174 = call-generic <vilib>:"NIMS_Complex To Real.vi"("A"=w426) -> ("Error Enum"=w420:T1, "Real(A)"=w425:dbl[][])  [unwired: 8 in, 1 out]
                  n175 = call-generic <vilib>:"NIMS_Get Scalar_w Error.vi"("A"=w425) -> ("Error Enum"=w419:T1, "Scalar"=w427:dbl)  [unwired: 8 in, 1 out]
                  n176 = call-generic <vilib>:"NIMS_Complex To Real.vi"("A"=w429) -> ("Error Enum"=w422:T1, "Real(A)"=w428:dbl[][])  [unwired: 8 in, 1 out]
                  n177 = call-generic <vilib>:"NIMS_Get Scalar_w Error.vi"("A"=w428) -> ("Error Enum"=w421:T1, "Scalar"=w430:dbl)  [unwired: 8 in, 1 out]
                  n178 = call-generic <vilib>:"NIMS_Get Row Vector_w Error - Matrix.vi"("A"=w433) -> ("Error Enum"=w424:T1, "Row Vector"=w432:T2[])  [unwired: 8 in, 1 out]
                  n179 = call <vilib>:"NIMS_CH_Character RV to String.vi"("Character array"=w432) -> ("String"=w434:string)  [unwired: 10 in]
                  n180 = call <vilib>:"NIMS_String to Enum.vi"("Input String"=w434, "Enum choices"=string[] ["minorder"] ("Enum Options")) -> ("Error Enum"=w423:T1, "Enum Index"=w435:i32)  [unwired: 8 in]
                  n181 = call <vilib>:"NIMS_DF_fir_halfband(m, f, ripple).vi"("ripple"=w427, "f"=w430, "flag"=w435) -> ("error"=w418:i32, "b"=w409:dbl[])  [unwired: 7 in]
                  n182 = Build Array(w412, w412, w412, w412, w412, w412, "fir_halfband") -> (w415:string[])
                  n183 = Build Array(w424, w423, w422, w421, w420, w419, w418) -> (w416:i32[])
                  n184 = call <vilib>:"NIMS_Create Error From Enums.vi"("Error Code"=bool[] [FALSE, FALSE, FALSE, FALSE, FALSE, FALSE, TRUE], "error in (no error)"=w414, "Line no"=w417, "Error Enums"=w416, "Function names"=w415) -> ("error out"=w410:errorcluster)  [unwired: 6 in]
                }
                frame "_Char:Character;;_Char:Character;" {
                  w439 = "fir_halfband"
                  n185 = call <vilib>:"NIMS_CH_Character 2D to U8 2D.vi"("Character 2D array"=w453) -> ("U8 2D array"=w452:u8[][])  [unwired: 10 in]
                  n186 = To Double Precision Float(number=w452) -> (double precision float=w451:dbl[][])
                  n187 = call-generic <vilib>:"NIMS_Get Scalar_w Error.vi"("A"=w451) -> ("Error Enum"=w446:T1, "Scalar"=w454:dbl)  [unwired: 8 in, 1 out]
                  n188 = call-generic <vilib>:"NIMS_Complex To Real.vi"("A"=w456) -> ("Error Enum"=w448:T1, "Real(A)"=w455:dbl[][])  [unwired: 8 in, 1 out]
                  n189 = call-generic <vilib>:"NIMS_Get Scalar_w Error.vi"("A"=w455) -> ("Error Enum"=w447:T1, "Scalar"=w457:dbl)  [unwired: 8 in, 1 out]
                  n190 = call-generic <vilib>:"NIMS_Get Row Vector_w Error - Matrix.vi"("A"=w460) -> ("Error Enum"=w450:T1, "Row Vector"=w459:T2[])  [unwired: 8 in, 1 out]
                  n191 = call <vilib>:"NIMS_CH_Character RV to String.vi"("Character array"=w459) -> ("String"=w461:string)  [unwired: 10 in]
                  n192 = call <vilib>:"NIMS_String to Enum.vi"("Input String"=w461, "Enum choices"=string[] ["minorder"] ("Enum Options")) -> ("Error Enum"=w449:T1, "Enum Index"=w462:i32)  [unwired: 8 in]
                  n193 = call <vilib>:"NIMS_DF_fir_halfband(m, f, ripple).vi"("ripple"=w454, "f"=w457, "flag"=w462) -> ("error"=w445:i32, "b"=w436:dbl[])  [unwired: 7 in]
                  n194 = Build Array(w439, w439, w439, w439, w439, "fir_halfband") -> (w442:string[])
                  n195 = Build Array(w450, w449, w448, w447, w446, w445) -> (w443:i32[])
                  n196 = call <vilib>:"NIMS_Create Error From Enums.vi"("Error Code"=bool[] [FALSE, FALSE, FALSE, FALSE, FALSE, TRUE], "error in (no error)"=w441, "Line no"=w444, "Error Enums"=w443, "Function names"=w442) -> ("error out"=w437:errorcluster)  [unwired: 6 in]
                }
              }
              n197 = Build Array(w325) -> (w324:dbl[][])
              n198 = To Double Precision Complex(1:w324) -> (0:w323:cdb[][])
              n199 = call-generic <vilib>:"NIMS_RunTimeType_From StrictType (excl LVString).vi"("Plug-In Name"="", "Data In"=w323) -> ("Data Out"=w321:variant)  [unwired: 2 in]
              n200 = Build Array(w321) -> (w320:variant[])
            }
          }
        }
        frame 4 {
          n201 = case shown="1" w463 {
            tunnel: [_ w475 w650] -> w469
            tunnel: w466 -> [w473 _ _]
            tunnel: w467 -> [w474 w501 w676]
            tunnel: w465 -> [w471 w499 w674]
            tunnel: [w470 w481 w656] -> w464
            tunnel: w468 -> [_ w502 w677]
            frame Default {
              n202 = call <vilib>:"Create Error.vi"("Function name"=w473, "error in (no error)"=w471, "Error Enum"=error."Wrong number of output arguments", "Line number"=w474) -> ("error out"=w470:errorcluster)  [unwired: 6 in, 1 out]
            }
            frame 0 {
              n203 = Index Array(array=w502) -> (element #1=w498:variant, element #2=w493:variant, element #3=w489:variant, element #4=w484:variant)  [unwired: 4 in]
              n204 = call <vilib>:"NIMS_RunTimeType_Get Case Value.vi"("Data In"=w484) -> ("Case Value"=w482:string)  [unwired: 9 in, 1 out]
              n205 = call <vilib>:"NIMS_CH_RunTimeType_To Character 2D.vi"("Variant"=w484) -> ("data"=w483:T2[][])  [unwired: 1 in]
              n206 = call <vilib>:"NIMS_RunTimeType_Get Case Value.vi"("Data In"=w489) -> ("Case Value"=w485:string)  [unwired: 9 in, 1 out]
              n207 = call <vilib>:"NIMS_CH_RunTimeType_To Character 2D.vi"("Variant"=w489) -> ("data"=w486:T2[][])  [unwired: 1 in]
              n208 = call-generic <vilib>:"NIMS_RunTimeType_To Numeric.vi"("DataType"=cdb[][] [], "Variant"=w489) -> ("data"=w487:cdb[][])  [unwired: 1 in]
              n209 = call <vilib>:"NIMS_RunTimeType_Get Case Value.vi"("Data In"=w493) -> ("Case Value"=w490:string)  [unwired: 9 in, 1 out]
              n210 = call-generic <vilib>:"NIMS_RunTimeType_To Numeric.vi"("DataType"=cdb[][] [], "Variant"=w493) -> ("data"=w491:cdb[][])  [unwired: 1 in]
              n211 = call <vilib>:"NIMS_RunTimeType_Get Case Value.vi"("Data In"=w498) -> ("Case Value"=w494:string)  [unwired: 9 in, 1 out]
              n212 = call <vilib>:"NIMS_CH_RunTimeType_To Character 2D.vi"("Variant"=w498) -> ("data"=w495:T2[][])  [unwired: 1 in]
              n213 = call-generic <vilib>:"NIMS_RunTimeType_To Numeric.vi"("DataType"=cdb[][] [], "Variant"=w498) -> ("data"=w496:cdb[][])  [unwired: 1 in]
              n214 = Concatenate Strings(w494, w490, w485, w482) -> (w500:string)
              n215 = case shown="\"_Char:Character;;_Char:Character;_Char:Character;\"" w500 {
                tunnel: w499 -> [w504 w513 w550 w587 w621]
                tunnel: [_ w508 w545 w582 w616] -> w480
                tunnel: [w503 w509 w546 w583 w617] -> w481
                tunnel: w496 -> [_ w542 w579 _ _]
                tunnel: w495 -> [_ _ _ w613 w647]
                tunnel: w491 -> [_ w536 w573 w609 w643]
                tunnel: w487 -> [_ w533 _ w606 _]
                tunnel: w486 -> [_ _ w570 _ w640]
                tunnel: w483 -> [_ w529 w565 w602 w635]
                tunnel: w501 -> [w507 w516 w553 w590 w624]
                frame Default {
                  n216 = call <vilib>:"Create Error.vi"("Function name"="fir_halfband", "error in (no error)"=w504, "Error Enum"=23, "Line number"=w507) -> ("error out"=w503:errorcluster)  [unwired: 6 in, 1 out]
                }
                frame ";;;_Char:Character;" {
                  w511 = "fir_halfband"
                  n217 = call-generic <vilib>:"NIMS_Get Row Vector_w Error - Matrix.vi"("A"=w529) -> ("Error Enum"=w519:T1, "Row Vector"=w528:T2[])  [unwired: 8 in, 1 out]
                  n218 = call <vilib>:"NIMS_CH_Character RV to String.vi"("Character array"=w528) -> ("String"=w530:string)  [unwired: 10 in]
                  n219 = call <vilib>:"NIMS_String to Enum.vi"("Input String"=w530, "Enum choices"=string[] ["high", "kaiser"] ("Enum Options")) -> ("Error Enum"=w518:T1, "Enum Index"=w531:i32)  [unwired: 8 in]
                  n220 = call-generic <vilib>:"NIMS_Complex To Real.vi"("A"=w533) -> ("Error Enum"=w521:T1, "Real(A)"=w532:dbl[][])  [unwired: 8 in, 1 out]
                  n221 = call-generic <vilib>:"NIMS_Get Scalar_w Error.vi"("A"=w532) -> ("Error Enum"=w520:T1, "Scalar"=w534:dbl)  [unwired: 8 in, 1 out]
                  n222 = call-generic <vilib>:"NIMS_Complex To Real.vi"("A"=w536) -> ("Error Enum"=w523:T1, "Real(A)"=w535:dbl[][])  [unwired: 8 in, 1 out]
                  n223 = call-generic <vilib>:"NIMS_Get Scalar_w Error.vi"("A"=w535) -> ("Error Enum"=w522:T1, "Scalar"=w537:dbl)  [unwired: 8 in, 1 out]
                  n224 = call-generic <vilib>:"NIMS_Complex To Real.vi"("A"=w542) -> ("Error Enum"=w526:T1, "Real(A)"=w541:dbl[][])  [unwired: 8 in, 1 out]
                  n225 = To Unsigned Byte Integer(number=w541) -> (unsigned 8bit integer=w540:u8[][])
                  n226 = call-generic <vilib>:"NIMS_Get Row Vector_w Error - Matrix.vi"("A"=w540) -> ("Error Enum"=w525:T1, "Row Vector"=w539:u8[])  [unwired: 8 in, 1 out]
                  n227 = Byte Array To String(unsigned byte array=w539) -> (string=w543:string)
                  n228 = call <vilib>:"NIMS_String to Enum.vi"("Input String"=w543, "Enum choices"=string[] ["minorder"] ("Enum Options")) -> ("Error Enum"=w524:T1, "Enum Index"=w544:i32)  [unwired: 8 in]
                  n229 = call <vilib>:"NIMS_DF_fir_halfband(m, f, ripple,kh).vi"("type"=w531, "ripple"=w534, "f"=w537, "flag"=w544) -> ("error"=w517:i32, "b"=w508:dbl[])  [unwired: 6 in]
                  n230 = Build Array(w511, w511, w511, w511, w511, w511, w511, w511, w511, "fir_halfband") -> (w514:string[])
                  n231 = Build Array(w526, w525, w524, w523, w522, w521, w520, w519, w518, w517) -> (w515:i32[])
                  n232 = call <vilib>:"NIMS_Create Error From Enums.vi"("Error Code"=bool[] [FALSE, FALSE, FALSE, FALSE, FALSE, FALSE, FALSE, FALSE, FALSE, TRUE], "error in (no error)"=w513, "Line no"=w516, "Error Enums"=w515, "Function names"=w514) -> ("error out"=w509:errorcluster)  [unwired: 6 in]
                }
                frame ";;_Char:Character;_Char:Character;" {
                  w548 = "fir_halfband"
                  n233 = call-generic <vilib>:"NIMS_Get Row Vector_w Error - Matrix.vi"("A"=w565) -> ("Error Enum"=w556:T1, "Row Vector"=w564:T2[])  [unwired: 8 in, 1 out]
                  n234 = call <vilib>:"NIMS_CH_Character RV to String.vi"("Character array"=w564) -> ("String"=w566:string)  [unwired: 10 in]
                  n235 = call <vilib>:"NIMS_String to Enum.vi"("Input String"=w566, "Enum choices"=string[] ["high", "kaiser"] ("Enum Options")) -> ("Error Enum"=w555:T1, "Enum Index"=w567:i32)  [unwired: 8 in]
                  n236 = call <vilib>:"NIMS_CH_Character 2D to U8 2D.vi"("Character 2D array"=w570) -> ("U8 2D array"=w569:u8[][])  [unwired: 10 in]
                  n237 = To Double Precision Float(number=w569) -> (double precision float=w568:dbl[][])
                  n238 = call-generic <vilib>:"NIMS_Get Scalar_w Error.vi"("A"=w568) -> ("Error Enum"=w557:T1, "Scalar"=w571:dbl)  [unwired: 8 in, 1 out]
                  n239 = call-generic <vilib>:"NIMS_Complex To Real.vi"("A"=w573) -> ("Error Enum"=w559:T1, "Real(A)"=w572:dbl[][])  [unwired: 8 in, 1 out]
                  n240 = call-generic <vilib>:"NIMS_Get Scalar_w Error.vi"("A"=w572) -> ("Error Enum"=w558:T1, "Scalar"=w574:dbl)  [unwired: 8 in, 1 out]
                  n241 = call-generic <vilib>:"NIMS_Complex To Real.vi"("A"=w579) -> ("Error Enum"=w562:T1, "Real(A)"=w578:dbl[][])  [unwired: 8 in, 1 out]
                  n242 = To Unsigned Byte Integer(number=w578) -> (unsigned 8bit integer=w577:u8[][])
                  n243 = call-generic <vilib>:"NIMS_Get Row Vector_w Error - Matrix.vi"("A"=w577) -> ("Error Enum"=w561:T1, "Row Vector"=w576:u8[])  [unwired: 8 in, 1 out]
                  n244 = Byte Array To String(unsigned byte array=w576) -> (string=w580:string)
                  n245 = call <vilib>:"NIMS_String to Enum.vi"("Input String"=w580, "Enum choices"=string[] ["minorder"] ("Enum Options")) -> ("Error Enum"=w560:T1, "Enum Index"=w581:i32)  [unwired: 8 in]
                  n246 = call <vilib>:"NIMS_DF_fir_halfband(m, f, ripple,kh).vi"("type"=w567, "ripple"=w571, "f"=w574, "flag"=w581) -> ("error"=w554:i32, "b"=w545:dbl[])  [unwired: 6 in]
                  n247 = Build Array(w548, w548, w548, w548, w548, w548, w548, w548, "fir_halfband") -> (w551:string[])
                  n248 = Build Array(w562, w561, w560, w559, w558, w557, w556, w555, w554) -> (w552:i32[])
                  n249 = call <vilib>:"NIMS_Create Error From Enums.vi"("Error Code"=bool[] [FALSE, FALSE, FALSE, FALSE, FALSE, FALSE, FALSE, FALSE, TRUE], "error in (no error)"=w550, "Line no"=w553, "Error Enums"=w552, "Function names"=w551) -> ("error out"=w546:errorcluster)  [unwired: 6 in]
                }
                frame "_Char:Character;;;_Char:Character;" {
                  w585 = "fir_halfband"
                  n250 = call-generic <vilib>:"NIMS_Get Row Vector_w Error - Matrix.vi"("A"=w602) -> ("Error Enum"=w593:T1, "Row Vector"=w601:T2[])  [unwired: 8 in, 1 out]
                  n251 = call <vilib>:"NIMS_CH_Character RV to String.vi"("Character array"=w601) -> ("String"=w603:string)  [unwired: 10 in]
                  n252 = call <vilib>:"NIMS_String to Enum.vi"("Input String"=w603, "Enum choices"=string[] ["high", "kaiser"] ("Enum Options")) -> ("Error Enum"=w592:T1, "Enum Index"=w604:i32)  [unwired: 8 in]
                  n253 = call-generic <vilib>:"NIMS_Complex To Real.vi"("A"=w606) -> ("Error Enum"=w595:T1, "Real(A)"=w605:dbl[][])  [unwired: 8 in, 1 out]
                  n254 = call-generic <vilib>:"NIMS_Get Scalar_w Error.vi"("A"=w605) -> ("Error Enum"=w594:T1, "Scalar"=w607:dbl)  [unwired: 8 in, 1 out]
                  n255 = call-generic <vilib>:"NIMS_Complex To Real.vi"("A"=w609) -> ("Error Enum"=w597:T1, "Real(A)"=w608:dbl[][])  [unwired: 8 in, 1 out]
                  n256 = call-generic <vilib>:"NIMS_Get Scalar_w Error.vi"("A"=w608) -> ("Error Enum"=w596:T1, "Scalar"=w610:dbl)  [unwired: 8 in, 1 out]
                  n257 = call-generic <vilib>:"NIMS_Get Row Vector_w Error - Matrix.vi"("A"=w613) -> ("Error Enum"=w599:T1, "Row Vector"=w612:T2[])  [unwired: 8 in, 1 out]
                  n258 = call <vilib>:"NIMS_CH_Character RV to String.vi"("Character array"=w612) -> ("String"=w614:string)  [unwired: 10 in]
                  n259 = call <vilib>:"NIMS_String to Enum.vi"("Input String"=w614, "Enum choices"=string[] ["minorder"] ("Enum Options")) -> ("Error Enum"=w598:T1, "Enum Index"=w615:i32)  [unwired: 8 in]
                  n260 = call <vilib>:"NIMS_DF_fir_halfband(m, f, ripple,kh).vi"("type"=w604, "ripple"=w607, "f"=w610, "flag"=w615) -> ("error"=w591:i32, "b"=w582:dbl[])  [unwired: 6 in]
                  n261 = Build Array(w585, w585, w585, w585, w585, w585, w585, w585, "fir_halfband") -> (w588:string[])
                  n262 = Build Array(w599, w598, w597, w596, w595, w594, w593, w592, w591) -> (w589:i32[])
                  n263 = call <vilib>:"NIMS_Create Error From Enums.vi"("Error Code"=bool[] [FALSE, FALSE, FALSE, FALSE, FALSE, FALSE, FALSE, FALSE, TRUE], "error in (no error)"=w587, "Line no"=w590, "Error Enums"=w589, "Function names"=w588) -> ("error out"=w583:errorcluster)  [unwired: 6 in]
                }
                frame "_Char:Character;;_Char:Character;_Char:Character;" {
                  w619 = "fir_halfband"
                  n264 = call-generic <vilib>:"NIMS_Get Row Vector_w Error - Matrix.vi"("A"=w635) -> ("Error Enum"=w627:T1, "Row Vector"=w634:T2[])  [unwired: 8 in, 1 out]
                  n265 = call <vilib>:"NIMS_CH_Character RV to String.vi"("Character array"=w634) -> ("String"=w636:string)  [unwired: 10 in]
                  n266 = call <vilib>:"NIMS_String to Enum.vi"("Input String"=w636, "Enum choices"=string[] ["high", "kaiser"] ("Enum Options")) -> ("Error Enum"=w626:T1, "Enum Index"=w637:i32)  [unwired: 8 in]
                  n267 = call <vilib>:"NIMS_CH_Character 2D to U8 2D.vi"("Character 2D array"=w640) -> ("U8 2D array"=w639:u8[][])  [unwired: 10 in]
                  n268 = To Double Precision Float(number=w639) -> (double precision float=w638:dbl[][])
                  n269 = call-generic <vilib>:"NIMS_Get Scalar_w Error.vi"("A"=w638) -> ("Error Enum"=w628:T1, "Scalar"=w641:dbl)  [unwired: 8 in, 1 out]
                  n270 = call-generic <vilib>:"NIMS_Complex To Real.vi"("A"=w643) -> ("Error Enum"=w630:T1, "Real(A)"=w642:dbl[][])  [unwired: 8 in, 1 out]
                  n271 = call-generic <vilib>:"NIMS_Get Scalar_w Error.vi"("A"=w642) -> ("Error Enum"=w629:T1, "Scalar"=w644:dbl)  [unwired: 8 in, 1 out]
                  n272 = call-generic <vilib>:"NIMS_Get Row Vector_w Error - Matrix.vi"("A"=w647) -> ("Error Enum"=w632:T1, "Row Vector"=w646:T2[])  [unwired: 8 in, 1 out]
                  n273 = call <vilib>:"NIMS_CH_Character RV to String.vi"("Character array"=w646) -> ("String"=w648:string)  [unwired: 10 in]
                  n274 = call <vilib>:"NIMS_String to Enum.vi"("Input String"=w648, "Enum choices"=string[] ["minorder"] ("Enum Options")) -> ("Error Enum"=w631:T1, "Enum Index"=w649:i32)  [unwired: 8 in]
                  n275 = call <vilib>:"NIMS_DF_fir_halfband(m, f, ripple,kh).vi"("type"=w637, "ripple"=w641, "f"=w644, "flag"=w649) -> ("error"=w625:i32, "b"=w616:dbl[])  [unwired: 6 in]
                  n276 = Build Array(w619, w619, w619, w619, w619, w619, w619, "fir_halfband") -> (w622:string[])
                  n277 = Build Array(w632, w631, w630, w629, w628, w627, w626, w625) -> (w623:i32[])
                  n278 = call <vilib>:"NIMS_Create Error From Enums.vi"("Error Code"=bool[] [FALSE, FALSE, FALSE, FALSE, FALSE, FALSE, FALSE, TRUE], "error in (no error)"=w621, "Line no"=w624, "Error Enums"=w623, "Function names"=w622) -> ("error out"=w617:errorcluster)  [unwired: 6 in]
                }
              }
              n279 = Build Array(w480) -> (w479:dbl[][])
              n280 = To Double Precision Complex(1:w479) -> (0:w478:cdb[][])
              n281 = call-generic <vilib>:"NIMS_RunTimeType_From StrictType (excl LVString).vi"("Plug-In Name"="", "Data In"=w478) -> ("Data Out"=w476:variant)  [unwired: 2 in]
              n282 = Build Array(w476) -> (w475:variant[])
            }
            frame 1 {
              n283 = Index Array(array=w677) -> (element #1=w673:variant, element #2=w668:variant, element #3=w664:variant, element #4=w659:variant)  [unwired: 4 in]
              n284 = call <vilib>:"NIMS_RunTimeType_Get Case Value.vi"("Data In"=w659) -> ("Case Value"=w657:string)  [unwired: 9 in, 1 out]
              n285 = call <vilib>:"NIMS_CH_RunTimeType_To Character 2D.vi"("Variant"=w659) -> ("data"=w658:T2[][])  [unwired: 1 in]
              n286 = call <vilib>:"NIMS_RunTimeType_Get Case Value.vi"("Data In"=w664) -> ("Case Value"=w660:string)  [unwired: 9 in, 1 out]
              n287 = call <vilib>:"NIMS_CH_RunTimeType_To Character 2D.vi"("Variant"=w664) -> ("data"=w661:T2[][])  [unwired: 1 in]
              n288 = call-generic <vilib>:"NIMS_RunTimeType_To Numeric.vi"("DataType"=cdb[][] [], "Variant"=w664) -> ("data"=w662:cdb[][])  [unwired: 1 in]
              n289 = call <vilib>:"NIMS_RunTimeType_Get Case Value.vi"("Data In"=w668) -> ("Case Value"=w665:string)  [unwired: 9 in, 1 out]
              n290 = call-generic <vilib>:"NIMS_RunTimeType_To Numeric.vi"("DataType"=cdb[][] [], "Variant"=w668) -> ("data"=w666:cdb[][])  [unwired: 1 in]
              n291 = call <vilib>:"NIMS_RunTimeType_Get Case Value.vi"("Data In"=w673) -> ("Case Value"=w669:string)  [unwired: 9 in, 1 out]
              n292 = call <vilib>:"NIMS_CH_RunTimeType_To Character 2D.vi"("Variant"=w673) -> ("data"=w670:T2[][])  [unwired: 1 in]
              n293 = call-generic <vilib>:"NIMS_RunTimeType_To Numeric.vi"("DataType"=cdb[][] [], "Variant"=w673) -> ("data"=w671:cdb[][])  [unwired: 1 in]
              n294 = Concatenate Strings(w669, w665, w660, w657) -> (w675:string)
              n295 = case shown="\"_Char:Character;;_Char:Character;_Char:Character;\"" w675 {
                tunnel: w674 -> [w679 w688 w725 w762 w796]
                tunnel: [_ w683 w720 w757 w791] -> w655
                tunnel: [w678 w684 w721 w758 w792] -> w656
                tunnel: w671 -> [_ w717 w754 _ _]
                tunnel: w670 -> [_ _ _ w788 w822]
                tunnel: w666 -> [_ w711 w748 w784 w818]
                tunnel: w662 -> [_ w708 _ w781 _]
                tunnel: w661 -> [_ _ w745 _ w815]
                tunnel: w658 -> [_ w704 w740 w777 w810]
                tunnel: w676 -> [w682 w691 w728 w765 w799]
                frame Default {
                  n296 = call <vilib>:"Create Error.vi"("Function name"="fir_halfband", "error in (no error)"=w679, "Error Enum"=23, "Line number"=w682) -> ("error out"=w678:errorcluster)  [unwired: 6 in, 1 out]
                }
                frame ";;;_Char:Character;" {
                  w686 = "fir_halfband"
                  n297 = call-generic <vilib>:"NIMS_Get Row Vector_w Error - Matrix.vi"("A"=w704) -> ("Error Enum"=w694:T1, "Row Vector"=w703:T2[])  [unwired: 8 in, 1 out]
                  n298 = call <vilib>:"NIMS_CH_Character RV to String.vi"("Character array"=w703) -> ("String"=w705:string)  [unwired: 10 in]
                  n299 = call <vilib>:"NIMS_String to Enum.vi"("Input String"=w705, "Enum choices"=string[] ["high", "kaiser"] ("Enum Options")) -> ("Error Enum"=w693:T1, "Enum Index"=w706:i32)  [unwired: 8 in]
                  n300 = call-generic <vilib>:"NIMS_Complex To Real.vi"("A"=w708) -> ("Error Enum"=w696:T1, "Real(A)"=w707:dbl[][])  [unwired: 8 in, 1 out]
                  n301 = call-generic <vilib>:"NIMS_Get Scalar_w Error.vi"("A"=w707) -> ("Error Enum"=w695:T1, "Scalar"=w709:dbl)  [unwired: 8 in, 1 out]
                  n302 = call-generic <vilib>:"NIMS_Complex To Real.vi"("A"=w711) -> ("Error Enum"=w698:T1, "Real(A)"=w710:dbl[][])  [unwired: 8 in, 1 out]
                  n303 = call-generic <vilib>:"NIMS_Get Scalar_w Error.vi"("A"=w710) -> ("Error Enum"=w697:T1, "Scalar"=w712:dbl)  [unwired: 8 in, 1 out]
                  n304 = call-generic <vilib>:"NIMS_Complex To Real.vi"("A"=w717) -> ("Error Enum"=w701:T1, "Real(A)"=w716:dbl[][])  [unwired: 8 in, 1 out]
                  n305 = To Unsigned Byte Integer(number=w716) -> (unsigned 8bit integer=w715:u8[][])
                  n306 = call-generic <vilib>:"NIMS_Get Row Vector_w Error - Matrix.vi"("A"=w715) -> ("Error Enum"=w700:T1, "Row Vector"=w714:u8[])  [unwired: 8 in, 1 out]
                  n307 = Byte Array To String(unsigned byte array=w714) -> (string=w718:string)
                  n308 = call <vilib>:"NIMS_String to Enum.vi"("Input String"=w718, "Enum choices"=string[] ["minorder"] ("Enum Options")) -> ("Error Enum"=w699:T1, "Enum Index"=w719:i32)  [unwired: 8 in]
                  n309 = call <vilib>:"NIMS_DF_fir_halfband(m, f, ripple,kh).vi"("type"=w706, "ripple"=w709, "f"=w712, "flag"=w719) -> ("error"=w692:i32, "b"=w683:dbl[])  [unwired: 6 in]
                  n310 = Build Array(w686, w686, w686, w686, w686, w686, w686, w686, w686, "fir_halfband") -> (w689:string[])
                  n311 = Build Array(w701, w700, w699, w698, w697, w696, w695, w694, w693, w692) -> (w690:i32[])
                  n312 = call <vilib>:"NIMS_Create Error From Enums.vi"("Error Code"=bool[] [FALSE, FALSE, FALSE, FALSE, FALSE, FALSE, FALSE, FALSE, FALSE, TRUE], "error in (no error)"=w688, "Line no"=w691, "Error Enums"=w690, "Function names"=w689) -> ("error out"=w684:errorcluster)  [unwired: 6 in]
                }
                frame ";;_Char:Character;_Char:Character;" {
                  w723 = "fir_halfband"
                  n313 = call-generic <vilib>:"NIMS_Get Row Vector_w Error - Matrix.vi"("A"=w740) -> ("Error Enum"=w731:T1, "Row Vector"=w739:T2[])  [unwired: 8 in, 1 out]
                  n314 = call <vilib>:"NIMS_CH_Character RV to String.vi"("Character array"=w739) -> ("String"=w741:string)  [unwired: 10 in]
                  n315 = call <vilib>:"NIMS_String to Enum.vi"("Input String"=w741, "Enum choices"=string[] ["high", "kaiser"] ("Enum Options")) -> ("Error Enum"=w730:T1, "Enum Index"=w742:i32)  [unwired: 8 in]
                  n316 = call <vilib>:"NIMS_CH_Character 2D to U8 2D.vi"("Character 2D array"=w745) -> ("U8 2D array"=w744:u8[][])  [unwired: 10 in]
                  n317 = To Double Precision Float(number=w744) -> (double precision float=w743:dbl[][])
                  n318 = call-generic <vilib>:"NIMS_Get Scalar_w Error.vi"("A"=w743) -> ("Error Enum"=w732:T1, "Scalar"=w746:dbl)  [unwired: 8 in, 1 out]
                  n319 = call-generic <vilib>:"NIMS_Complex To Real.vi"("A"=w748) -> ("Error Enum"=w734:T1, "Real(A)"=w747:dbl[][])  [unwired: 8 in, 1 out]
                  n320 = call-generic <vilib>:"NIMS_Get Scalar_w Error.vi"("A"=w747) -> ("Error Enum"=w733:T1, "Scalar"=w749:dbl)  [unwired: 8 in, 1 out]
                  n321 = call-generic <vilib>:"NIMS_Complex To Real.vi"("A"=w754) -> ("Error Enum"=w737:T1, "Real(A)"=w753:dbl[][])  [unwired: 8 in, 1 out]
                  n322 = To Unsigned Byte Integer(number=w753) -> (unsigned 8bit integer=w752:u8[][])
                  n323 = call-generic <vilib>:"NIMS_Get Row Vector_w Error - Matrix.vi"("A"=w752) -> ("Error Enum"=w736:T1, "Row Vector"=w751:u8[])  [unwired: 8 in, 1 out]
                  n324 = Byte Array To String(unsigned byte array=w751) -> (string=w755:string)
                  n325 = call <vilib>:"NIMS_String to Enum.vi"("Input String"=w755, "Enum choices"=string[] ["minorder"] ("Enum Options")) -> ("Error Enum"=w735:T1, "Enum Index"=w756:i32)  [unwired: 8 in]
                  n326 = call <vilib>:"NIMS_DF_fir_halfband(m, f, ripple,kh).vi"("type"=w742, "ripple"=w746, "f"=w749, "flag"=w756) -> ("error"=w729:i32, "b"=w720:dbl[])  [unwired: 6 in]
                  n327 = Build Array(w723, w723, w723, w723, w723, w723, w723, w723, "fir_halfband") -> (w726:string[])
                  n328 = Build Array(w737, w736, w735, w734, w733, w732, w731, w730, w729) -> (w727:i32[])
                  n329 = call <vilib>:"NIMS_Create Error From Enums.vi"("Error Code"=bool[] [FALSE, FALSE, FALSE, FALSE, FALSE, FALSE, FALSE, FALSE, TRUE], "error in (no error)"=w725, "Line no"=w728, "Error Enums"=w727, "Function names"=w726) -> ("error out"=w721:errorcluster)  [unwired: 6 in]
                }
                frame "_Char:Character;;;_Char:Character;" {
                  w760 = "fir_halfband"
                  n330 = call-generic <vilib>:"NIMS_Get Row Vector_w Error - Matrix.vi"("A"=w777) -> ("Error Enum"=w768:T1, "Row Vector"=w776:T2[])  [unwired: 8 in, 1 out]
                  n331 = call <vilib>:"NIMS_CH_Character RV to String.vi"("Character array"=w776) -> ("String"=w778:string)  [unwired: 10 in]
                  n332 = call <vilib>:"NIMS_String to Enum.vi"("Input String"=w778, "Enum choices"=string[] ["high", "kaiser"] ("Enum Options")) -> ("Error Enum"=w767:T1, "Enum Index"=w779:i32)  [unwired: 8 in]
                  n333 = call-generic <vilib>:"NIMS_Complex To Real.vi"("A"=w781) -> ("Error Enum"=w770:T1, "Real(A)"=w780:dbl[][])  [unwired: 8 in, 1 out]
                  n334 = call-generic <vilib>:"NIMS_Get Scalar_w Error.vi"("A"=w780) -> ("Error Enum"=w769:T1, "Scalar"=w782:dbl)  [unwired: 8 in, 1 out]
                  n335 = call-generic <vilib>:"NIMS_Complex To Real.vi"("A"=w784) -> ("Error Enum"=w772:T1, "Real(A)"=w783:dbl[][])  [unwired: 8 in, 1 out]
                  n336 = call-generic <vilib>:"NIMS_Get Scalar_w Error.vi"("A"=w783) -> ("Error Enum"=w771:T1, "Scalar"=w785:dbl)  [unwired: 8 in, 1 out]
                  n337 = call-generic <vilib>:"NIMS_Get Row Vector_w Error - Matrix.vi"("A"=w788) -> ("Error Enum"=w774:T1, "Row Vector"=w787:T2[])  [unwired: 8 in, 1 out]
                  n338 = call <vilib>:"NIMS_CH_Character RV to String.vi"("Character array"=w787) -> ("String"=w789:string)  [unwired: 10 in]
                  n339 = call <vilib>:"NIMS_String to Enum.vi"("Input String"=w789, "Enum choices"=string[] ["minorder"] ("Enum Options")) -> ("Error Enum"=w773:T1, "Enum Index"=w790:i32)  [unwired: 8 in]
                  n340 = call <vilib>:"NIMS_DF_fir_halfband(m, f, ripple,kh).vi"("type"=w779, "ripple"=w782, "f"=w785, "flag"=w790) -> ("error"=w766:i32, "b"=w757:dbl[])  [unwired: 6 in]
                  n341 = Build Array(w760, w760, w760, w760, w760, w760, w760, w760, "fir_halfband") -> (w763:string[])
                  n342 = Build Array(w774, w773, w772, w771, w770, w769, w768, w767, w766) -> (w764:i32[])
                  n343 = call <vilib>:"NIMS_Create Error From Enums.vi"("Error Code"=bool[] [FALSE, FALSE, FALSE, FALSE, FALSE, FALSE, FALSE, FALSE, TRUE], "error in (no error)"=w762, "Line no"=w765, "Error Enums"=w764, "Function names"=w763) -> ("error out"=w758:errorcluster)  [unwired: 6 in]
                }
                frame "_Char:Character;;_Char:Character;_Char:Character;" {
                  w794 = "fir_halfband"
                  n344 = call-generic <vilib>:"NIMS_Get Row Vector_w Error - Matrix.vi"("A"=w810) -> ("Error Enum"=w802:T1, "Row Vector"=w809:T2[])  [unwired: 8 in, 1 out]
                  n345 = call <vilib>:"NIMS_CH_Character RV to String.vi"("Character array"=w809) -> ("String"=w811:string)  [unwired: 10 in]
                  n346 = call <vilib>:"NIMS_String to Enum.vi"("Input String"=w811, "Enum choices"=string[] ["high", "kaiser"] ("Enum Options")) -> ("Error Enum"=w801:T1, "Enum Index"=w812:i32)  [unwired: 8 in]
                  n347 = call <vilib>:"NIMS_CH_Character 2D to U8 2D.vi"("Character 2D array"=w815) -> ("U8 2D array"=w814:u8[][])  [unwired: 10 in]
                  n348 = To Double Precision Float(number=w814) -> (double precision float=w813:dbl[][])
                  n349 = call-generic <vilib>:"NIMS_Get Scalar_w Error.vi"("A"=w813) -> ("Error Enum"=w803:T1, "Scalar"=w816:dbl)  [unwired: 8 in, 1 out]
                  n350 = call-generic <vilib>:"NIMS_Complex To Real.vi"("A"=w818) -> ("Error Enum"=w805:T1, "Real(A)"=w817:dbl[][])  [unwired: 8 in, 1 out]
                  n351 = call-generic <vilib>:"NIMS_Get Scalar_w Error.vi"("A"=w817) -> ("Error Enum"=w804:T1, "Scalar"=w819:dbl)  [unwired: 8 in, 1 out]
                  n352 = call-generic <vilib>:"NIMS_Get Row Vector_w Error - Matrix.vi"("A"=w822) -> ("Error Enum"=w807:T1, "Row Vector"=w821:T2[])  [unwired: 8 in, 1 out]
                  n353 = call <vilib>:"NIMS_CH_Character RV to String.vi"("Character array"=w821) -> ("String"=w823:string)  [unwired: 10 in]
                  n354 = call <vilib>:"NIMS_String to Enum.vi"("Input String"=w823, "Enum choices"=string[] ["minorder"] ("Enum Options")) -> ("Error Enum"=w806:T1, "Enum Index"=w824:i32)  [unwired: 8 in]
                  n355 = call <vilib>:"NIMS_DF_fir_halfband(m, f, ripple,kh).vi"("type"=w812, "ripple"=w816, "f"=w819, "flag"=w824) -> ("error"=w800:i32, "b"=w791:dbl[])  [unwired: 6 in]
                  n356 = Build Array(w794, w794, w794, w794, w794, w794, w794, "fir_halfband") -> (w797:string[])
                  n357 = Build Array(w807, w806, w805, w804, w803, w802, w801, w800) -> (w798:i32[])
                  n358 = call <vilib>:"NIMS_Create Error From Enums.vi"("Error Code"=bool[] [FALSE, FALSE, FALSE, FALSE, FALSE, FALSE, FALSE, TRUE], "error in (no error)"=w796, "Line no"=w799, "Error Enums"=w798, "Function names"=w797) -> ("error out"=w792:errorcluster)  [unwired: 6 in]
                }
              }
              n359 = Build Array(w655) -> (w654:dbl[][])
              n360 = To Double Precision Complex(1:w654) -> (0:w653:cdb[][])
              n361 = call-generic <vilib>:"NIMS_RunTimeType_From StrictType (excl LVString).vi"("Plug-In Name"="", "Data In"=w653) -> ("Data Out"=w651:variant)  [unwired: 2 in]
              n362 = Build Array(w651) -> (w650:variant[])
            }
          }
        }
        frame 5 {
          n363 = case shown="1" w825 {
            tunnel: [_ w837 w1043] -> w831
            tunnel: w828 -> [w835 _ _]
            tunnel: w829 -> [w836 w866 w1072]
            tunnel: w827 -> [w833 w864 w1070]
            tunnel: [w832 w843 w1049] -> w826
            tunnel: w830 -> [_ w867 w1073]
            frame Default {
              n364 = call <vilib>:"Create Error.vi"("Function name"=w835, "error in (no error)"=w833, "Error Enum"=error."Wrong number of output arguments", "Line number"=w836) -> ("error out"=w832:errorcluster)  [unwired: 6 in, 1 out]
            }
            frame 0 {
              n365 = Index Array(array=w867) -> (element #1=w863:variant, element #2=w858:variant, element #3=w854:variant, element #4=w849:variant, element #5=w846:variant)  [unwired: 5 in]
              n366 = call <vilib>:"NIMS_RunTimeType_Get Case Value.vi"("Data In"=w846) -> ("Case Value"=w844:string)  [unwired: 9 in, 1 out]
              n367 = call <vilib>:"NIMS_CH_RunTimeType_To Character 2D.vi"("Variant"=w846) -> ("data"=w845:T2[][])  [unwired: 1 in]
              n368 = call <vilib>:"NIMS_RunTimeType_Get Case Value.vi"("Data In"=w849) -> ("Case Value"=w847:string)  [unwired: 9 in, 1 out]
              n369 = call <vilib>:"NIMS_CH_RunTimeType_To Character 2D.vi"("Variant"=w849) -> ("data"=w848:T2[][])  [unwired: 1 in]
              n370 = call <vilib>:"NIMS_RunTimeType_Get Case Value.vi"("Data In"=w854) -> ("Case Value"=w850:string)  [unwired: 9 in, 1 out]
              n371 = call <vilib>:"NIMS_CH_RunTimeType_To Character 2D.vi"("Variant"=w854) -> ("data"=w851:T2[][])  [unwired: 1 in]
              n372 = call-generic <vilib>:"NIMS_RunTimeType_To Numeric.vi"("DataType"=cdb[][] [], "Variant"=w854) -> ("data"=w852:cdb[][])  [unwired: 1 in]
              n373 = call <vilib>:"NIMS_RunTimeType_Get Case Value.vi"("Data In"=w858) -> ("Case Value"=w855:string)  [unwired: 9 in, 1 out]
              n374 = call-generic <vilib>:"NIMS_RunTimeType_To Numeric.vi"("DataType"=cdb[][] [], "Variant"=w858) -> ("data"=w856:cdb[][])  [unwired: 1 in]
              n375 = call <vilib>:"NIMS_RunTimeType_Get Case Value.vi"("Data In"=w863) -> ("Case Value"=w859:string)  [unwired: 9 in, 1 out]
              n376 = call <vilib>:"NIMS_CH_RunTimeType_To Character 2D.vi"("Variant"=w863) -> ("data"=w860:T2[][])  [unwired: 1 in]
              n377 = call-generic <vilib>:"NIMS_RunTimeType_To Numeric.vi"("DataType"=cdb[][] [], "Variant"=w863) -> ("data"=w861:cdb[][])  [unwired: 1 in]
              n378 = Concatenate Strings(w859, w855, w850, w847, w844) -> (w865:string)
              n379 = case shown="\"_Char:Character;;_Char:Character;_Char:Character;_Char:Character;\"" w865 {
                tunnel: w864 -> [w869 w878 w922 w966 w1007]
                tunnel: [_ w873 w917 w961 w1002] -> w842
                tunnel: [w868 w874 w918 w962 w1003] -> w843
                tunnel: w861 -> [_ w914 w958 _ _]
                tunnel: w860 -> [_ _ _ w999 w1040]
                tunnel: w856 -> [_ w908 w952 w995 w1036]
                tunnel: w852 -> [_ w905 _ w992 _]
                tunnel: w851 -> [_ _ w949 _ w1033]
                tunnel: w848 -> [_ w901 w944 w988 w1028]
                tunnel: w845 -> [_ w896 w939 w983 w1023]
                tunnel: w866 -> [w872 w881 w925 w969 w1010]
                frame Default {
                  n380 = call <vilib>:"Create Error.vi"("Function name"="fir_halfband", "error in (no error)"=w869, "Error Enum"=23, "Line number"=w872) -> ("error out"=w868:errorcluster)  [unwired: 6 in, 1 out]
                }
                frame ";;;_Char:Character;_Char:Character;" {
                  w876 = "fir_halfband"
                  n381 = call-generic <vilib>:"NIMS_Get Row Vector_w Error - Matrix.vi"("A"=w896) -> ("Error Enum"=w884:T1, "Row Vector"=w895:T2[])  [unwired: 8 in, 1 out]
                  n382 = call <vilib>:"NIMS_CH_Character RV to String.vi"("Character array"=w895) -> ("String"=w897:string)  [unwired: 10 in]
                  n383 = call <vilib>:"NIMS_String to Enum.vi"("Input String"=w897, "Enum choices"=string[] ["high"] ("Enum Options")) -> ("Error Enum"=w883:T1, "Enum Index"=w898:i32)  [unwired: 8 in]
                  n384 = call-generic <vilib>:"NIMS_Get Row Vector_w Error - Matrix.vi"("A"=w901) -> ("Error Enum"=w886:T1, "Row Vector"=w900:T2[])  [unwired: 8 in, 1 out]
                  n385 = call <vilib>:"NIMS_CH_Character RV to String.vi"("Character array"=w900) -> ("String"=w902:string)  [unwired: 10 in]
                  n386 = call <vilib>:"NIMS_String to Enum.vi"("Input String"=w902, "Enum choices"=string[] ["kaiser"] ("Enum Options")) -> ("Error Enum"=w885:T1, "Enum Index"=w903:i32)  [unwired: 8 in]
                  n387 = call-generic <vilib>:"NIMS_Complex To Real.vi"("A"=w905) -> ("Error Enum"=w888:T1, "Real(A)"=w904:dbl[][])  [unwired: 8 in, 1 out]
                  n388 = call-generic <vilib>:"NIMS_Get Scalar_w Error.vi"("A"=w904) -> ("Error Enum"=w887:T1, "Scalar"=w906:dbl)  [unwired: 8 in, 1 out]
                  n389 = call-generic <vilib>:"NIMS_Complex To Real.vi"("A"=w908) -> ("Error Enum"=w890:T1, "Real(A)"=w907:dbl[][])  [unwired: 8 in, 1 out]
                  n390 = call-generic <vilib>:"NIMS_Get Scalar_w Error.vi"("A"=w907) -> ("Error Enum"=w889:T1, "Scalar"=w909:dbl)  [unwired: 8 in, 1 out]
                  n391 = call-generic <vilib>:"NIMS_Complex To Real.vi"("A"=w914) -> ("Error Enum"=w893:T1, "Real(A)"=w913:dbl[][])  [unwired: 8 in, 1 out]
                  n392 = To Unsigned Byte Integer(number=w913) -> (unsigned 8bit integer=w912:u8[][])
                  n393 = call-generic <vilib>:"NIMS_Get Row Vector_w Error - Matrix.vi"("A"=w912) -> ("Error Enum"=w892:T1, "Row Vector"=w911:u8[])  [unwired: 8 in, 1 out]
                  n394 = Byte Array To String(unsigned byte array=w911) -> (string=w915:string)
                  n395 = call <vilib>:"NIMS_String to Enum.vi"("Input String"=w915, "Enum choices"=string[] ["minorder"] ("Enum Options")) -> ("Error Enum"=w891:T1, "Enum Index"=w916:i32)  [unwired: 8 in]
                  n396 = call <vilib>:"NIMS_DF_fir_halfband(m, f, ripple,k,h).vi"("type"=w898, "method"=w903, "ripple"=w906, "f"=w909, "flag"=w916) -> ("error"=w882:i32, "b"=w873:dbl[])  [unwired: 5 in]
                  n397 = Build Array(w876, w876, w876, w876, w876, w876, w876, w876, w876, w876, w876, "fir_halfband") -> (w879:string[])
                  n398 = Build Array(w893, w892, w891, w890, w889, w888, w887, w886, w885, w884, w883, w882) -> (w880:i32[])
                  n399 = call <vilib>:"NIMS_Create Error From Enums.vi"("Error Code"=bool[] [FALSE, FALSE, FALSE, FALSE, FALSE, FALSE, FALSE, FALSE, FALSE, FALSE, FALSE, TRUE], "error in (no error)"=w878, "Line no"=w881, "Error Enums"=w880, "Function names"=w879) -> ("error out"=w874:errorcluster)  [unwired: 6 in]
                }
                frame ";;_Char:Character;_Char:Character;_Char:Character;" {
                  w920 = "fir_halfband"
                  n400 = call-generic <vilib>:"NIMS_Get Row Vector_w Error - Matrix.vi"("A"=w939) -> ("Error Enum"=w928:T1, "Row Vector"=w938:T2[])  [unwired: 8 in, 1 out]
                  n401 = call <vilib>:"NIMS_CH_Character RV to String.vi"("Character array"=w938) -> ("String"=w940:string)  [unwired: 10 in]
                  n402 = call <vilib>:"NIMS_String to Enum.vi"("Input String"=w940, "Enum choices"=string[] ["high"] ("Enum Options")) -> ("Error Enum"=w927:T1, "Enum Index"=w941:i32)  [unwired: 8 in]
                  n403 = call-generic <vilib>:"NIMS_Get Row Vector_w Error - Matrix.vi"("A"=w944) -> ("Error Enum"=w930:T1, "Row Vector"=w943:T2[])  [unwired: 8 in, 1 out]
                  n404 = call <vilib>:"NIMS_CH_Character RV to String.vi"("Character array"=w943) -> ("String"=w945:string)  [unwired: 10 in]
                  n405 = call <vilib>:"NIMS_String to Enum.vi"("Input String"=w945, "Enum choices"=string[] ["kaiser"] ("Enum Options")) -> ("Error Enum"=w929:T1, "Enum Index"=w946:i32)  [unwired: 8 in]
                  n406 = call <vilib>:"NIMS_CH_Character 2D to U8 2D.vi"("Character 2D array"=w949) -> ("U8 2D array"=w948:u8[][])  [unwired: 10 in]
                  n407 = To Double Precision Float(number=w948) -> (double precision float=w947:dbl[][])
                  n408 = call-generic <vilib>:"NIMS_Get Scalar_w Error.vi"("A"=w947) -> ("Error Enum"=w931:T1, "Scalar"=w950:dbl)  [unwired: 8 in, 1 out]
                  n409 = call-generic <vilib>:"NIMS_Complex To Real.vi"("A"=w952) -> ("Error Enum"=w933:T1, "Real(A)"=w951:dbl[][])  [unwired: 8 in, 1 out]
                  n410 = call-generic <vilib>:"NIMS_Get Scalar_w Error.vi"("A"=w951) -> ("Error Enum"=w932:T1, "Scalar"=w953:dbl)  [unwired: 8 in, 1 out]
                  n411 = call-generic <vilib>:"NIMS_Complex To Real.vi"("A"=w958) -> ("Error Enum"=w936:T1, "Real(A)"=w957:dbl[][])  [unwired: 8 in, 1 out]
                  n412 = To Unsigned Byte Integer(number=w957) -> (unsigned 8bit integer=w956:u8[][])
                  n413 = call-generic <vilib>:"NIMS_Get Row Vector_w Error - Matrix.vi"("A"=w956) -> ("Error Enum"=w935:T1, "Row Vector"=w955:u8[])  [unwired: 8 in, 1 out]
                  n414 = Byte Array To String(unsigned byte array=w955) -> (string=w959:string)
                  n415 = call <vilib>:"NIMS_String to Enum.vi"("Input String"=w959, "Enum choices"=string[] ["minorder"] ("Enum Options")) -> ("Error Enum"=w934:T1, "Enum Index"=w960:i32)  [unwired: 8 in]
                  n416 = call <vilib>:"NIMS_DF_fir_halfband(m, f, ripple,k,h).vi"("type"=w941, "method"=w946, "ripple"=w950, "f"=w953, "flag"=w960) -> ("error"=w926:i32, "b"=w917:dbl[])  [unwired: 5 in]
                  n417 = Build Array(w920, w920, w920, w920, w920, w920, w920, w920, w920, w920, "fir_halfband") -> (w923:string[])
                  n418 = Build Array(w936, w935, w934, w933, w932, w931, w930, w929, w928, w927, w926) -> (w924:i32[])
                  n419 = call <vilib>:"NIMS_Create Error From Enums.vi"("Error Code"=bool[] [FALSE, FALSE, FALSE, FALSE, FALSE, FALSE, FALSE, FALSE, FALSE, FALSE, TRUE], "error in (no error)"=w922, "Line no"=w925, "Error Enums"=w924, "Function names"=w923) -> ("error out"=w918:errorcluster)  [unwired: 6 in]
                }
                frame "_Char:Character;;;_Char:Character;_Char:Character;" {
                  w964 = "fir_halfband"
                  n420 = call-generic <vilib>:"NIMS_Get Row Vector_w Error - Matrix.vi"("A"=w983) -> ("Error Enum"=w972:T1, "Row Vector"=w982:T2[])  [unwired: 8 in, 1 out]
                  n421 = call <vilib>:"NIMS_CH_Character RV to String.vi"("Character array"=w982) -> ("String"=w984:string)  [unwired: 10 in]
                  n422 = call <vilib>:"NIMS_String to Enum.vi"("Input String"=w984, "Enum choices"=string[] ["high"] ("Enum Options")) -> ("Error Enum"=w971:T1, "Enum Index"=w985:i32)  [unwired: 8 in]
                  n423 = call-generic <vilib>:"NIMS_Get Row Vector_w Error - Matrix.vi"("A"=w988) -> ("Error Enum"=w974:T1, "Row Vector"=w987:T2[])  [unwired: 8 in, 1 out]
                  n424 = call <vilib>:"NIMS_CH_Character RV to String.vi"("Character array"=w987) -> ("String"=w989:string)  [unwired: 10 in]
                  n425 = call <vilib>:"NIMS_String to Enum.vi"("Input String"=w989, "Enum choices"=string[] ["kaiser"] ("Enum Options")) -> ("Error Enum"=w973:T1, "Enum Index"=w990:i32)  [unwired: 8 in]
                  n426 = call-generic <vilib>:"NIMS_Complex To Real.vi"("A"=w992) -> ("Error Enum"=w976:T1, "Real(A)"=w991:dbl[][])  [unwired: 8 in, 1 out]
                  n427 = call-generic <vilib>:"NIMS_Get Scalar_w Error.vi"("A"=w991) -> ("Error Enum"=w975:T1, "Scalar"=w993:dbl)  [unwired: 8 in, 1 out]
                  n428 = call-generic <vilib>:"NIMS_Complex To Real.vi"("A"=w995) -> ("Error Enum"=w978:T1, "Real(A)"=w994:dbl[][])  [unwired: 8 in, 1 out]
                  n429 = call-generic <vilib>:"NIMS_Get Scalar_w Error.vi"("A"=w994) -> ("Error Enum"=w977:T1, "Scalar"=w996:dbl)  [unwired: 8 in, 1 out]
                  n430 = call-generic <vilib>:"NIMS_Get Row Vector_w Error - Matrix.vi"("A"=w999) -> ("Error Enum"=w980:T1, "Row Vector"=w998:T2[])  [unwired: 8 in, 1 out]
                  n431 = call <vilib>:"NIMS_CH_Character RV to String.vi"("Character array"=w998) -> ("String"=w1000:string)  [unwired: 10 in]
                  n432 = call <vilib>:"NIMS_String to Enum.vi"("Input String"=w1000, "Enum choices"=string[] ["minorder"] ("Enum Options")) -> ("Error Enum"=w979:T1, "Enum Index"=w1001:i32)  [unwired: 8 in]
                  n433 = call <vilib>:"NIMS_DF_fir_halfband(m, f, ripple,k,h).vi"("type"=w985, "method"=w990, "ripple"=w993, "f"=w996, "flag"=w1001) -> ("error"=w970:i32, "b"=w961:dbl[])  [unwired: 5 in]
                  n434 = Build Array(w964, w964, w964, w964, w964, w964, w964, w964, w964, w964, "fir_halfband") -> (w967:string[])
                  n435 = Build Array(w980, w979, w978, w977, w976, w975, w974, w973, w972, w971, w970) -> (w968:i32[])
                  n436 = call <vilib>:"NIMS_Create Error From Enums.vi"("Error Code"=bool[] [FALSE, FALSE, FALSE, FALSE, FALSE, FALSE, FALSE, FALSE, FALSE, FALSE, TRUE], "error in (no error)"=w966, "Line no"=w969, "Error Enums"=w968, "Function names"=w967) -> ("error out"=w962:errorcluster)  [unwired: 6 in]
                }
                frame "_Char:Character;;_Char:Character;_Char:Character;_Char:Character;" {
                  w1005 = "fir_halfband"
                  n437 = call-generic <vilib>:"NIMS_Get Row Vector_w Error - Matrix.vi"("A"=w1023) -> ("Error Enum"=w1013:T1, "Row Vector"=w1022:T2[])  [unwired: 8 in, 1 out]
                  n438 = call <vilib>:"NIMS_CH_Character RV to String.vi"("Character array"=w1022) -> ("String"=w1024:string)  [unwired: 10 in]
                  n439 = call <vilib>:"NIMS_String to Enum.vi"("Input String"=w1024, "Enum choices"=string[] ["high"] ("Enum Options")) -> ("Error Enum"=w1012:T1, "Enum Index"=w1025:i32)  [unwired: 8 in]
                  n440 = call-generic <vilib>:"NIMS_Get Row Vector_w Error - Matrix.vi"("A"=w1028) -> ("Error Enum"=w1015:T1, "Row Vector"=w1027:T2[])  [unwired: 8 in, 1 out]
                  n441 = call <vilib>:"NIMS_CH_Character RV to String.vi"("Character array"=w1027) -> ("String"=w1029:string)  [unwired: 10 in]
                  n442 = call <vilib>:"NIMS_String to Enum.vi"("Input String"=w1029, "Enum choices"=string[] ["kaiser"] ("Enum Options")) -> ("Error Enum"=w1014:T1, "Enum Index"=w1030:i32)  [unwired: 8 in]
                  n443 = call <vilib>:"NIMS_CH_Character 2D to U8 2D.vi"("Character 2D array"=w1033) -> ("U8 2D array"=w1032:u8[][])  [unwired: 10 in]
                  n444 = To Double Precision Float(number=w1032) -> (double precision float=w1031:dbl[][])
                  n445 = call-generic <vilib>:"NIMS_Get Scalar_w Error.vi"("A"=w1031) -> ("Error Enum"=w1016:T1, "Scalar"=w1034:dbl)  [unwired: 8 in, 1 out]
                  n446 = call-generic <vilib>:"NIMS_Complex To Real.vi"("A"=w1036) -> ("Error Enum"=w1018:T1, "Real(A)"=w1035:dbl[][])  [unwired: 8 in, 1 out]
                  n447 = call-generic <vilib>:"NIMS_Get Scalar_w Error.vi"("A"=w1035) -> ("Error Enum"=w1017:T1, "Scalar"=w1037:dbl)  [unwired: 8 in, 1 out]
                  n448 = call-generic <vilib>:"NIMS_Get Row Vector_w Error - Matrix.vi"("A"=w1040) -> ("Error Enum"=w1020:T1, "Row Vector"=w1039:T2[])  [unwired: 8 in, 1 out]
                  n449 = call <vilib>:"NIMS_CH_Character RV to String.vi"("Character array"=w1039) -> ("String"=w1041:string)  [unwired: 10 in]
                  n450 = call <vilib>:"NIMS_String to Enum.vi"("Input String"=w1041, "Enum choices"=string[] ["minorder"] ("Enum Options")) -> ("Error Enum"=w1019:T1, "Enum Index"=w1042:i32)  [unwired: 8 in]
                  n451 = call <vilib>:"NIMS_DF_fir_halfband(m, f, ripple,k,h).vi"("type"=w1025, "method"=w1030, "ripple"=w1034, "f"=w1037, "flag"=w1042) -> ("error"=w1011:i32, "b"=w1002:dbl[])  [unwired: 5 in]
                  n452 = Build Array(w1005, w1005, w1005, w1005, w1005, w1005, w1005, w1005, w1005, "fir_halfband") -> (w1008:string[])
                  n453 = Build Array(w1020, w1019, w1018, w1017, w1016, w1015, w1014, w1013, w1012, w1011) -> (w1009:i32[])
                  n454 = call <vilib>:"NIMS_Create Error From Enums.vi"("Error Code"=bool[] [FALSE, FALSE, FALSE, FALSE, FALSE, FALSE, FALSE, FALSE, FALSE, TRUE], "error in (no error)"=w1007, "Line no"=w1010, "Error Enums"=w1009, "Function names"=w1008) -> ("error out"=w1003:errorcluster)  [unwired: 6 in]
                }
              }
              n455 = Build Array(w842) -> (w841:dbl[][])
              n456 = To Double Precision Complex(1:w841) -> (0:w840:cdb[][])
              n457 = call-generic <vilib>:"NIMS_RunTimeType_From StrictType (excl LVString).vi"("Plug-In Name"="", "Data In"=w840) -> ("Data Out"=w838:variant)  [unwired: 2 in]
              n458 = Build Array(w838) -> (w837:variant[])
            }
            frame 1 {
              n459 = Index Array(array=w1073) -> (element #1=w1069:variant, element #2=w1064:variant, element #3=w1060:variant, element #4=w1055:variant, element #5=w1052:variant)  [unwired: 5 in]
              n460 = call <vilib>:"NIMS_RunTimeType_Get Case Value.vi"("Data In"=w1052) -> ("Case Value"=w1050:string)  [unwired: 9 in, 1 out]
              n461 = call <vilib>:"NIMS_CH_RunTimeType_To Character 2D.vi"("Variant"=w1052) -> ("data"=w1051:T2[][])  [unwired: 1 in]
              n462 = call <vilib>:"NIMS_RunTimeType_Get Case Value.vi"("Data In"=w1055) -> ("Case Value"=w1053:string)  [unwired: 9 in, 1 out]
              n463 = call <vilib>:"NIMS_CH_RunTimeType_To Character 2D.vi"("Variant"=w1055) -> ("data"=w1054:T2[][])  [unwired: 1 in]
              n464 = call <vilib>:"NIMS_RunTimeType_Get Case Value.vi"("Data In"=w1060) -> ("Case Value"=w1056:string)  [unwired: 9 in, 1 out]
              n465 = call <vilib>:"NIMS_CH_RunTimeType_To Character 2D.vi"("Variant"=w1060) -> ("data"=w1057:T2[][])  [unwired: 1 in]
              n466 = call-generic <vilib>:"NIMS_RunTimeType_To Numeric.vi"("DataType"=cdb[][] [], "Variant"=w1060) -> ("data"=w1058:cdb[][])  [unwired: 1 in]
              n467 = call <vilib>:"NIMS_RunTimeType_Get Case Value.vi"("Data In"=w1064) -> ("Case Value"=w1061:string)  [unwired: 9 in, 1 out]
              n468 = call-generic <vilib>:"NIMS_RunTimeType_To Numeric.vi"("DataType"=cdb[][] [], "Variant"=w1064) -> ("data"=w1062:cdb[][])  [unwired: 1 in]
              n469 = call <vilib>:"NIMS_RunTimeType_Get Case Value.vi"("Data In"=w1069) -> ("Case Value"=w1065:string)  [unwired: 9 in, 1 out]
              n470 = call <vilib>:"NIMS_CH_RunTimeType_To Character 2D.vi"("Variant"=w1069) -> ("data"=w1066:T2[][])  [unwired: 1 in]
              n471 = call-generic <vilib>:"NIMS_RunTimeType_To Numeric.vi"("DataType"=cdb[][] [], "Variant"=w1069) -> ("data"=w1067:cdb[][])  [unwired: 1 in]
              n472 = Concatenate Strings(w1065, w1061, w1056, w1053, w1050) -> (w1071:string)
              n473 = case shown="\"_Char:Character;;_Char:Character;_Char:Character;_Char:Character;\"" w1071 {
                tunnel: w1070 -> [w1075 w1084 w1128 w1172 w1213]
                tunnel: [_ w1079 w1123 w1167 w1208] -> w1048
                tunnel: [w1074 w1080 w1124 w1168 w1209] -> w1049
                tunnel: w1067 -> [_ w1120 w1164 _ _]
                tunnel: w1066 -> [_ _ _ w1205 w1246]
                tunnel: w1062 -> [_ w1114 w1158 w1201 w1242]
                tunnel: w1058 -> [_ w1111 _ w1198 _]
                tunnel: w1057 -> [_ _ w1155 _ w1239]
                tunnel: w1054 -> [_ w1107 w1150 w1194 w1234]
                tunnel: w1051 -> [_ w1102 w1145 w1189 w1229]
                tunnel: w1072 -> [w1078 w1087 w1131 w1175 w1216]
                frame Default {
                  n474 = call <vilib>:"Create Error.vi"("Function name"="fir_halfband", "error in (no error)"=w1075, "Error Enum"=23, "Line number"=w1078) -> ("error out"=w1074:errorcluster)  [unwired: 6 in, 1 out]
                }
                frame ";;;_Char:Character;_Char:Character;" {
                  w1082 = "fir_halfband"
                  n475 = call-generic <vilib>:"NIMS_Get Row Vector_w Error - Matrix.vi"("A"=w1102) -> ("Error Enum"=w1090:T1, "Row Vector"=w1101:T2[])  [unwired: 8 in, 1 out]
                  n476 = call <vilib>:"NIMS_CH_Character RV to String.vi"("Character array"=w1101) -> ("String"=w1103:string)  [unwired: 10 in]
                  n477 = call <vilib>:"NIMS_String to Enum.vi"("Input String"=w1103, "Enum choices"=string[] ["high"] ("Enum Options")) -> ("Error Enum"=w1089:T1, "Enum Index"=w1104:i32)  [unwired: 8 in]
                  n478 = call-generic <vilib>:"NIMS_Get Row Vector_w Error - Matrix.vi"("A"=w1107) -> ("Error Enum"=w1092:T1, "Row Vector"=w1106:T2[])  [unwired: 8 in, 1 out]
                  n479 = call <vilib>:"NIMS_CH_Character RV to String.vi"("Character array"=w1106) -> ("String"=w1108:string)  [unwired: 10 in]
                  n480 = call <vilib>:"NIMS_String to Enum.vi"("Input String"=w1108, "Enum choices"=string[] ["kaiser"] ("Enum Options")) -> ("Error Enum"=w1091:T1, "Enum Index"=w1109:i32)  [unwired: 8 in]
                  n481 = call-generic <vilib>:"NIMS_Complex To Real.vi"("A"=w1111) -> ("Error Enum"=w1094:T1, "Real(A)"=w1110:dbl[][])  [unwired: 8 in, 1 out]
                  n482 = call-generic <vilib>:"NIMS_Get Scalar_w Error.vi"("A"=w1110) -> ("Error Enum"=w1093:T1, "Scalar"=w1112:dbl)  [unwired: 8 in, 1 out]
                  n483 = call-generic <vilib>:"NIMS_Complex To Real.vi"("A"=w1114) -> ("Error Enum"=w1096:T1, "Real(A)"=w1113:dbl[][])  [unwired: 8 in, 1 out]
                  n484 = call-generic <vilib>:"NIMS_Get Scalar_w Error.vi"("A"=w1113) -> ("Error Enum"=w1095:T1, "Scalar"=w1115:dbl)  [unwired: 8 in, 1 out]
                  n485 = call-generic <vilib>:"NIMS_Complex To Real.vi"("A"=w1120) -> ("Error Enum"=w1099:T1, "Real(A)"=w1119:dbl[][])  [unwired: 8 in, 1 out]
                  n486 = To Unsigned Byte Integer(number=w1119) -> (unsigned 8bit integer=w1118:u8[][])
                  n487 = call-generic <vilib>:"NIMS_Get Row Vector_w Error - Matrix.vi"("A"=w1118) -> ("Error Enum"=w1098:T1, "Row Vector"=w1117:u8[])  [unwired: 8 in, 1 out]
                  n488 = Byte Array To String(unsigned byte array=w1117) -> (string=w1121:string)
                  n489 = call <vilib>:"NIMS_String to Enum.vi"("Input String"=w1121, "Enum choices"=string[] ["minorder"] ("Enum Options")) -> ("Error Enum"=w1097:T1, "Enum Index"=w1122:i32)  [unwired: 8 in]
                  n490 = call <vilib>:"NIMS_DF_fir_halfband(m, f, ripple,k,h).vi"("type"=w1104, "method"=w1109, "ripple"=w1112, "f"=w1115, "flag"=w1122) -> ("error"=w1088:i32, "b"=w1079:dbl[])  [unwired: 5 in]
                  n491 = Build Array(w1082, w1082, w1082, w1082, w1082, w1082, w1082, w1082, w1082, w1082, w1082, "fir_halfband") -> (w1085:string[])
                  n492 = Build Array(w1099, w1098, w1097, w1096, w1095, w1094, w1093, w1092, w1091, w1090, w1089, w1088) -> (w1086:i32[])
                  n493 = call <vilib>:"NIMS_Create Error From Enums.vi"("Error Code"=bool[] [FALSE, FALSE, FALSE, FALSE, FALSE, FALSE, FALSE, FALSE, FALSE, FALSE, FALSE, TRUE], "error in (no error)"=w1084, "Line no"=w1087, "Error Enums"=w1086, "Function names"=w1085) -> ("error out"=w1080:errorcluster)  [unwired: 6 in]
                }
                frame ";;_Char:Character;_Char:Character;_Char:Character;" {
                  w1126 = "fir_halfband"
                  n494 = call-generic <vilib>:"NIMS_Get Row Vector_w Error - Matrix.vi"("A"=w1145) -> ("Error Enum"=w1134:T1, "Row Vector"=w1144:T2[])  [unwired: 8 in, 1 out]
                  n495 = call <vilib>:"NIMS_CH_Character RV to String.vi"("Character array"=w1144) -> ("String"=w1146:string)  [unwired: 10 in]
                  n496 = call <vilib>:"NIMS_String to Enum.vi"("Input String"=w1146, "Enum choices"=string[] ["high"] ("Enum Options")) -> ("Error Enum"=w1133:T1, "Enum Index"=w1147:i32)  [unwired: 8 in]
                  n497 = call-generic <vilib>:"NIMS_Get Row Vector_w Error - Matrix.vi"("A"=w1150) -> ("Error Enum"=w1136:T1, "Row Vector"=w1149:T2[])  [unwired: 8 in, 1 out]
                  n498 = call <vilib>:"NIMS_CH_Character RV to String.vi"("Character array"=w1149) -> ("String"=w1151:string)  [unwired: 10 in]
                  n499 = call <vilib>:"NIMS_String to Enum.vi"("Input String"=w1151, "Enum choices"=string[] ["kaiser"] ("Enum Options")) -> ("Error Enum"=w1135:T1, "Enum Index"=w1152:i32)  [unwired: 8 in]
                  n500 = call <vilib>:"NIMS_CH_Character 2D to U8 2D.vi"("Character 2D array"=w1155) -> ("U8 2D array"=w1154:u8[][])  [unwired: 10 in]
                  n501 = To Double Precision Float(number=w1154) -> (double precision float=w1153:dbl[][])
                  n502 = call-generic <vilib>:"NIMS_Get Scalar_w Error.vi"("A"=w1153) -> ("Error Enum"=w1137:T1, "Scalar"=w1156:dbl)  [unwired: 8 in, 1 out]
                  n503 = call-generic <vilib>:"NIMS_Complex To Real.vi"("A"=w1158) -> ("Error Enum"=w1139:T1, "Real(A)"=w1157:dbl[][])  [unwired: 8 in, 1 out]
                  n504 = call-generic <vilib>:"NIMS_Get Scalar_w Error.vi"("A"=w1157) -> ("Error Enum"=w1138:T1, "Scalar"=w1159:dbl)  [unwired: 8 in, 1 out]
                  n505 = call-generic <vilib>:"NIMS_Complex To Real.vi"("A"=w1164) -> ("Error Enum"=w1142:T1, "Real(A)"=w1163:dbl[][])  [unwired: 8 in, 1 out]
                  n506 = To Unsigned Byte Integer(number=w1163) -> (unsigned 8bit integer=w1162:u8[][])
                  n507 = call-generic <vilib>:"NIMS_Get Row Vector_w Error - Matrix.vi"("A"=w1162) -> ("Error Enum"=w1141:T1, "Row Vector"=w1161:u8[])  [unwired: 8 in, 1 out]
                  n508 = Byte Array To String(unsigned byte array=w1161) -> (string=w1165:string)
                  n509 = call <vilib>:"NIMS_String to Enum.vi"("Input String"=w1165, "Enum choices"=string[] ["minorder"] ("Enum Options")) -> ("Error Enum"=w1140:T1, "Enum Index"=w1166:i32)  [unwired: 8 in]
                  n510 = call <vilib>:"NIMS_DF_fir_halfband(m, f, ripple,k,h).vi"("type"=w1147, "method"=w1152, "ripple"=w1156, "f"=w1159, "flag"=w1166) -> ("error"=w1132:i32, "b"=w1123:dbl[])  [unwired: 5 in]
                  n511 = Build Array(w1126, w1126, w1126, w1126, w1126, w1126, w1126, w1126, w1126, w1126, "fir_halfband") -> (w1129:string[])
                  n512 = Build Array(w1142, w1141, w1140, w1139, w1138, w1137, w1136, w1135, w1134, w1133, w1132) -> (w1130:i32[])
                  n513 = call <vilib>:"NIMS_Create Error From Enums.vi"("Error Code"=bool[] [FALSE, FALSE, FALSE, FALSE, FALSE, FALSE, FALSE, FALSE, FALSE, FALSE, TRUE], "error in (no error)"=w1128, "Line no"=w1131, "Error Enums"=w1130, "Function names"=w1129) -> ("error out"=w1124:errorcluster)  [unwired: 6 in]
                }
                frame "_Char:Character;;;_Char:Character;_Char:Character;" {
                  w1170 = "fir_halfband"
                  n514 = call-generic <vilib>:"NIMS_Get Row Vector_w Error - Matrix.vi"("A"=w1189) -> ("Error Enum"=w1178:T1, "Row Vector"=w1188:T2[])  [unwired: 8 in, 1 out]
                  n515 = call <vilib>:"NIMS_CH_Character RV to String.vi"("Character array"=w1188) -> ("String"=w1190:string)  [unwired: 10 in]
                  n516 = call <vilib>:"NIMS_String to Enum.vi"("Input String"=w1190, "Enum choices"=string[] ["high"] ("Enum Options")) -> ("Error Enum"=w1177:T1, "Enum Index"=w1191:i32)  [unwired: 8 in]
                  n517 = call-generic <vilib>:"NIMS_Get Row Vector_w Error - Matrix.vi"("A"=w1194) -> ("Error Enum"=w1180:T1, "Row Vector"=w1193:T2[])  [unwired: 8 in, 1 out]
                  n518 = call <vilib>:"NIMS_CH_Character RV to String.vi"("Character array"=w1193) -> ("String"=w1195:string)  [unwired: 10 in]
                  n519 = call <vilib>:"NIMS_String to Enum.vi"("Input String"=w1195, "Enum choices"=string[] ["kaiser"] ("Enum Options")) -> ("Error Enum"=w1179:T1, "Enum Index"=w1196:i32)  [unwired: 8 in]
                  n520 = call-generic <vilib>:"NIMS_Complex To Real.vi"("A"=w1198) -> ("Error Enum"=w1182:T1, "Real(A)"=w1197:dbl[][])  [unwired: 8 in, 1 out]
                  n521 = call-generic <vilib>:"NIMS_Get Scalar_w Error.vi"("A"=w1197) -> ("Error Enum"=w1181:T1, "Scalar"=w1199:dbl)  [unwired: 8 in, 1 out]
                  n522 = call-generic <vilib>:"NIMS_Complex To Real.vi"("A"=w1201) -> ("Error Enum"=w1184:T1, "Real(A)"=w1200:dbl[][])  [unwired: 8 in, 1 out]
                  n523 = call-generic <vilib>:"NIMS_Get Scalar_w Error.vi"("A"=w1200) -> ("Error Enum"=w1183:T1, "Scalar"=w1202:dbl)  [unwired: 8 in, 1 out]
                  n524 = call-generic <vilib>:"NIMS_Get Row Vector_w Error - Matrix.vi"("A"=w1205) -> ("Error Enum"=w1186:T1, "Row Vector"=w1204:T2[])  [unwired: 8 in, 1 out]
                  n525 = call <vilib>:"NIMS_CH_Character RV to String.vi"("Character array"=w1204) -> ("String"=w1206:string)  [unwired: 10 in]
                  n526 = call <vilib>:"NIMS_String to Enum.vi"("Input String"=w1206, "Enum choices"=string[] ["minorder"] ("Enum Options")) -> ("Error Enum"=w1185:T1, "Enum Index"=w1207:i32)  [unwired: 8 in]
                  n527 = call <vilib>:"NIMS_DF_fir_halfband(m, f, ripple,k,h).vi"("type"=w1191, "method"=w1196, "ripple"=w1199, "f"=w1202, "flag"=w1207) -> ("error"=w1176:i32, "b"=w1167:dbl[])  [unwired: 5 in]
                  n528 = Build Array(w1170, w1170, w1170, w1170, w1170, w1170, w1170, w1170, w1170, w1170, "fir_halfband") -> (w1173:string[])
                  n529 = Build Array(w1186, w1185, w1184, w1183, w1182, w1181, w1180, w1179, w1178, w1177, w1176) -> (w1174:i32[])
                  n530 = call <vilib>:"NIMS_Create Error From Enums.vi"("Error Code"=bool[] [FALSE, FALSE, FALSE, FALSE, FALSE, FALSE, FALSE, FALSE, FALSE, FALSE, TRUE], "error in (no error)"=w1172, "Line no"=w1175, "Error Enums"=w1174, "Function names"=w1173) -> ("error out"=w1168:errorcluster)  [unwired: 6 in]
                }
                frame "_Char:Character;;_Char:Character;_Char:Character;_Char:Character;" {
                  w1211 = "fir_halfband"
                  n531 = call-generic <vilib>:"NIMS_Get Row Vector_w Error - Matrix.vi"("A"=w1229) -> ("Error Enum"=w1219:T1, "Row Vector"=w1228:T2[])  [unwired: 8 in, 1 out]
                  n532 = call <vilib>:"NIMS_CH_Character RV to String.vi"("Character array"=w1228) -> ("String"=w1230:string)  [unwired: 10 in]
                  n533 = call <vilib>:"NIMS_String to Enum.vi"("Input String"=w1230, "Enum choices"=string[] ["high"] ("Enum Options")) -> ("Error Enum"=w1218:T1, "Enum Index"=w1231:i32)  [unwired: 8 in]
                  n534 = call-generic <vilib>:"NIMS_Get Row Vector_w Error - Matrix.vi"("A"=w1234) -> ("Error Enum"=w1221:T1, "Row Vector"=w1233:T2[])  [unwired: 8 in, 1 out]
                  n535 = call <vilib>:"NIMS_CH_Character RV to String.vi"("Character array"=w1233) -> ("String"=w1235:string)  [unwired: 10 in]
                  n536 = call <vilib>:"NIMS_String to Enum.vi"("Input String"=w1235, "Enum choices"=string[] ["kaiser"] ("Enum Options")) -> ("Error Enum"=w1220:T1, "Enum Index"=w1236:i32)  [unwired: 8 in]
                  n537 = call <vilib>:"NIMS_CH_Character 2D to U8 2D.vi"("Character 2D array"=w1239) -> ("U8 2D array"=w1238:u8[][])  [unwired: 10 in]
                  n538 = To Double Precision Float(number=w1238) -> (double precision float=w1237:dbl[][])
                  n539 = call-generic <vilib>:"NIMS_Get Scalar_w Error.vi"("A"=w1237) -> ("Error Enum"=w1222:T1, "Scalar"=w1240:dbl)  [unwired: 8 in, 1 out]
                  n540 = call-generic <vilib>:"NIMS_Complex To Real.vi"("A"=w1242) -> ("Error Enum"=w1224:T1, "Real(A)"=w1241:dbl[][])  [unwired: 8 in, 1 out]
                  n541 = call-generic <vilib>:"NIMS_Get Scalar_w Error.vi"("A"=w1241) -> ("Error Enum"=w1223:T1, "Scalar"=w1243:dbl)  [unwired: 8 in, 1 out]
                  n542 = call-generic <vilib>:"NIMS_Get Row Vector_w Error - Matrix.vi"("A"=w1246) -> ("Error Enum"=w1226:T1, "Row Vector"=w1245:T2[])  [unwired: 8 in, 1 out]
                  n543 = call <vilib>:"NIMS_CH_Character RV to String.vi"("Character array"=w1245) -> ("String"=w1247:string)  [unwired: 10 in]
                  n544 = call <vilib>:"NIMS_String to Enum.vi"("Input String"=w1247, "Enum choices"=string[] ["minorder"] ("Enum Options")) -> ("Error Enum"=w1225:T1, "Enum Index"=w1248:i32)  [unwired: 8 in]
                  n545 = call <vilib>:"NIMS_DF_fir_halfband(m, f, ripple,k,h).vi"("type"=w1231, "method"=w1236, "ripple"=w1240, "f"=w1243, "flag"=w1248) -> ("error"=w1217:i32, "b"=w1208:dbl[])  [unwired: 5 in]
                  n546 = Build Array(w1211, w1211, w1211, w1211, w1211, w1211, w1211, w1211, w1211, "fir_halfband") -> (w1214:string[])
                  n547 = Build Array(w1226, w1225, w1224, w1223, w1222, w1221, w1220, w1219, w1218, w1217) -> (w1215:i32[])
                  n548 = call <vilib>:"NIMS_Create Error From Enums.vi"("Error Code"=bool[] [FALSE, FALSE, FALSE, FALSE, FALSE, FALSE, FALSE, FALSE, FALSE, TRUE], "error in (no error)"=w1213, "Line no"=w1216, "Error Enums"=w1215, "Function names"=w1214) -> ("error out"=w1209:errorcluster)  [unwired: 6 in]
                }
              }
              n549 = Build Array(w1048) -> (w1047:dbl[][])
              n550 = To Double Precision Complex(1:w1047) -> (0:w1046:cdb[][])
              n551 = call-generic <vilib>:"NIMS_RunTimeType_From StrictType (excl LVString).vi"("Plug-In Name"="", "Data In"=w1046) -> ("Data Out"=w1044:variant)  [unwired: 2 in]
              n552 = Build Array(w1044) -> (w1043:variant[])
            }
          }
        }
      }
    }
    frame Error {
    }
  }
  "error out" <- w3
  "[funct(A)]" <- w4
